vi "Marvin.vi"() -> ()   [LabVIEW 2017]
uses:
  Marvin ATP Remake 1.5.18/PCAN_Driver/ControlCAN.llb/CAN Channel.ctl
  Marvin ATP Remake 6.5.18 - Copy/PCAN_Driver/ControlCAN.llb/DevType.ctl
  Marvin ATP Remake 6.5.18/PCAN_Driver/ControlCAN.llb/VCI_INIT_CONFIG.ctl
  Marvin ATP Remake 6.5.18/PCAN_Driver/ControlCAN.llb/InitFlag.ctl
  Marvin ATP Remake 6.5.18/PCAN_Driver/ControlCAN.llb/Fliter.ctl
  Marvin ATP Remake 6.5.18/PCAN_Driver/ControlCAN.llb/Mode.ctl
  <vilib>/Utility/miscctls.llb/LVMinMaxIncTypeDef.ctl
  PCAN_Driver/ControlCAN.llb/VCI_CAN_OBJ.ctl
  PCAN_Driver/ControlCAN.lvlib
panel:
  in  "Graph Plot":bool
  in  "Get":bool
  in  "Set":bool
  out "Array 2":dbl[](array[numeric])
  in  "Clear Data Array":bool
  in  "PlayPause Data Array":bool
  out "CAN Data":cluster{"Frame Data":u64, "Frame ID":u32}[](array[cluster]) {"Frame ID" format="%.0x"; "Frame Data" format="%016x"}
  out "Waveform Chart":dbl(graph)
  in  "Help Button":bool
  in  "Clear Monitor":bool
  out "Array":u64[][](array[numeric]) format="%016x"
  out "Ambient Over temp":bool
  out "Ambient Sensor temp":bool
  out "Ambient Temperature":dbl
  in  "Motor Over Temp":bool
  in  "Speed control":bool
  out "Unit Adress":string
  in  "Serial Send":bool
  in  "Index":u16(ring) items=["1"=1, "2"=2, "3"=3]
  out "read buffer":string
  in  "SetGet":enum16{"Get", "Set"}(ring)
  in  "Function":T1(ring)
  in  "Value":dbl
  in  "Value 1/2":enum16{"1", "2"}(ring)
  out "Msg Count":u32
  in  "Param to Set":u16(ring) items=["EBAY 5F"=95, "AHU 3F"=63, "AHU 2F"=47]
  out "UUT":u8
  out "Horizontal Progress Bar":i32(slide) min=0 max=48 scale=0.0..50.0
  in  "Set Param.":bool
  in  "Serial Monitor":bool caption="Graph Button"
  in  "Serial Com":bool
  in  "VISA resource name":refnum<visa-resource-name>="COM6"
  out "Serial Status":bool
  in  "Graph Button":bool
  in  "Refresh Button":bool
  out "Data Send":u64 format="%016x"
  in  "Motor Speed RPM":u16
  out "Under voltage/Over voltage":bool
  out "Speed error":bool
  out "Derated drive temp":bool
  out "Motor Over temperature":bool
  out "Commutation err":bool
  out "Motor Sensor temp Fauilre":bool
  out "Drive Over temperature":bool
  out "Drive Sensor temp Failure":bool
  out "Motor Phase Current RMS":dbl
  out "ECS State":u16
  out "Motor Speed RPM":dbl
  out "Motor Stator Temp.":dbl
  out "Power transistor Heat sink Temp.":dbl
  out "DC Current":dbl
  out "DC Voltage":dbl
  in  "Can Send":bool
  in  "Stop":bool
  out "Config_CANAT":T8 {"DevType" items=["USB-CAN"=3, "USB-CAN2"=4]; "CanIndex" items=["通道1", "通道2"]; "VCI_INIT_CONFIG"."Fliter" items=["接收所有类型"=3, "只接收标准帧"=4, "只接收扩展帧"=7]; "VCI_INIT_CONFIG"."Mode" items=["正常工作", "自测模式（环回）", "仅侦听模式"]; "VCI_INIT_CONFIG"."InitFlag" items=["使用Flash参数", "使用界面设置参数"]}
  in  "Channel 2":T3 caption="Channel" items=["Channel 1", "Channel 2"]
  out "CAN Status":bool
  out "Driver Version":string
  out "Hall Sensor Fault":bool
  out "Motor Phase Current":dbl
  in  "Motor Phase Current":u16
  # "ver 1.7e"
  # "Marvin"
  # "REDLER TECHNOLOGIES LTD"
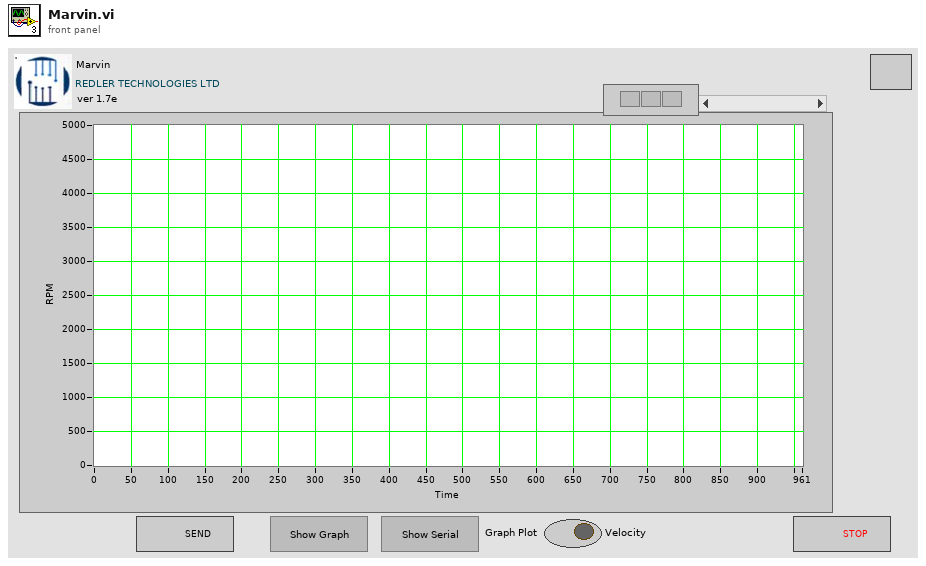
[diagram p1: front panel]
types:
  T1 = enum16{"Enable Conf. EP=1", "Serial Number", "Temperature", "Unit Adress", "Calibration", "Velocity", "Version"}
  T2 = typedef "ControlCAN.lvlib/DevType.ctl" = u32
  T3 = typedef "ControlCAN.lvlib/CAN Channel.ctl" = u32
  T4 = typedef "ControlCAN.lvlib/VCI_INIT_CONFIG.ctl" = cluster{"AccCode":u32, "AccMask":u32, "InitFlag":T5, "Fliter":T6, "Timing0":u8, "Timing1":u8, "Mode":T7}
  T5 = typedef "ControlCAN.lvlib/InitFlag.ctl" = u32
  T6 = typedef "ControlCAN.lvlib/Fliter.ctl" = u8
  T7 = typedef "ControlCAN.lvlib/Mode.ctl" = u8
  T8 = cluster{"DevType":T2, "DevIndex":u32, "CanIndex":T3, "VCI_INIT_CONFIG":T4}
  T9 = cluster{"ID":u32, "MSGTYPE":u8, "LEN":u8, "aDATA":u8[]}[]
  T10 = cluster{"ID":u32, "MSGTYPE":u8, "LEN":u8, "aDATA":u8[]}
  T11 = enum8{"Enabled", "Disabled", "Disabled and Grayed Out"}
  T12 = typedef "LVMinMaxIncTypeDef.ctl" = cluster{"Minimum":dbl, "Maximum":dbl, "Increment":dbl}
  T13 = enum32{"Invalid", "Standard", "Closed", "Hidden", "Minimized", "Maximized"}
  T14 = typedef "ControlCAN.lvlib/VCI_CAN_OBJ.ctl" = cluster{"ID":u32, "TimeStamp":u32, "TimeFlag":u8, "SendType":u8, "RemoteFlag":u8, "ExternFlag":u8, "DataLen":u8, "Data":u8[], "Reserved":u8[]}
  T15 = cluster{"Type":enum16{"接收", "发送"}, "Channel":T3, "Time":timestamp, "VCI_CAN_OBJ":T14}[]
  T16 = cluster{"Type":enum16{"接收", "发送"}, "Channel":T3, "Time":timestamp, "VCI_CAN_OBJ":T14}
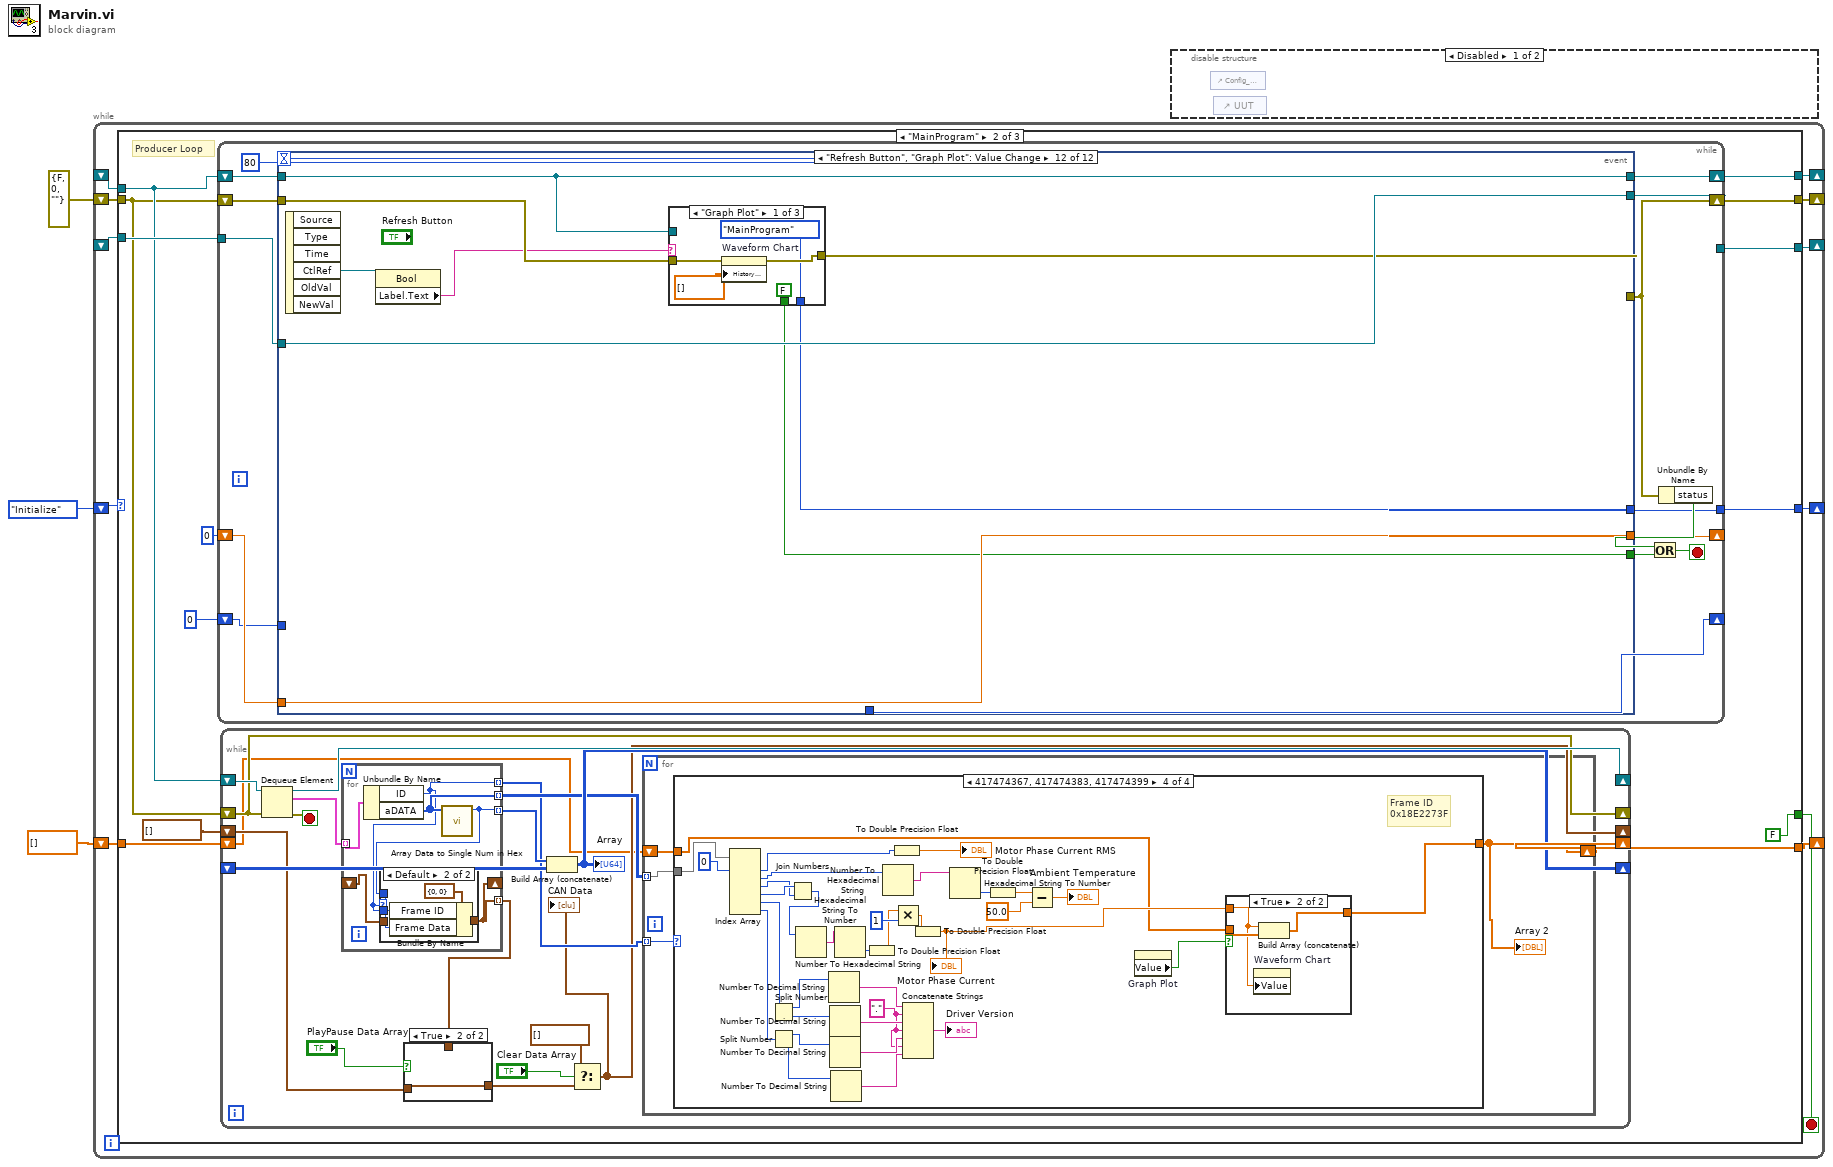
[diagram p0: block diagram]
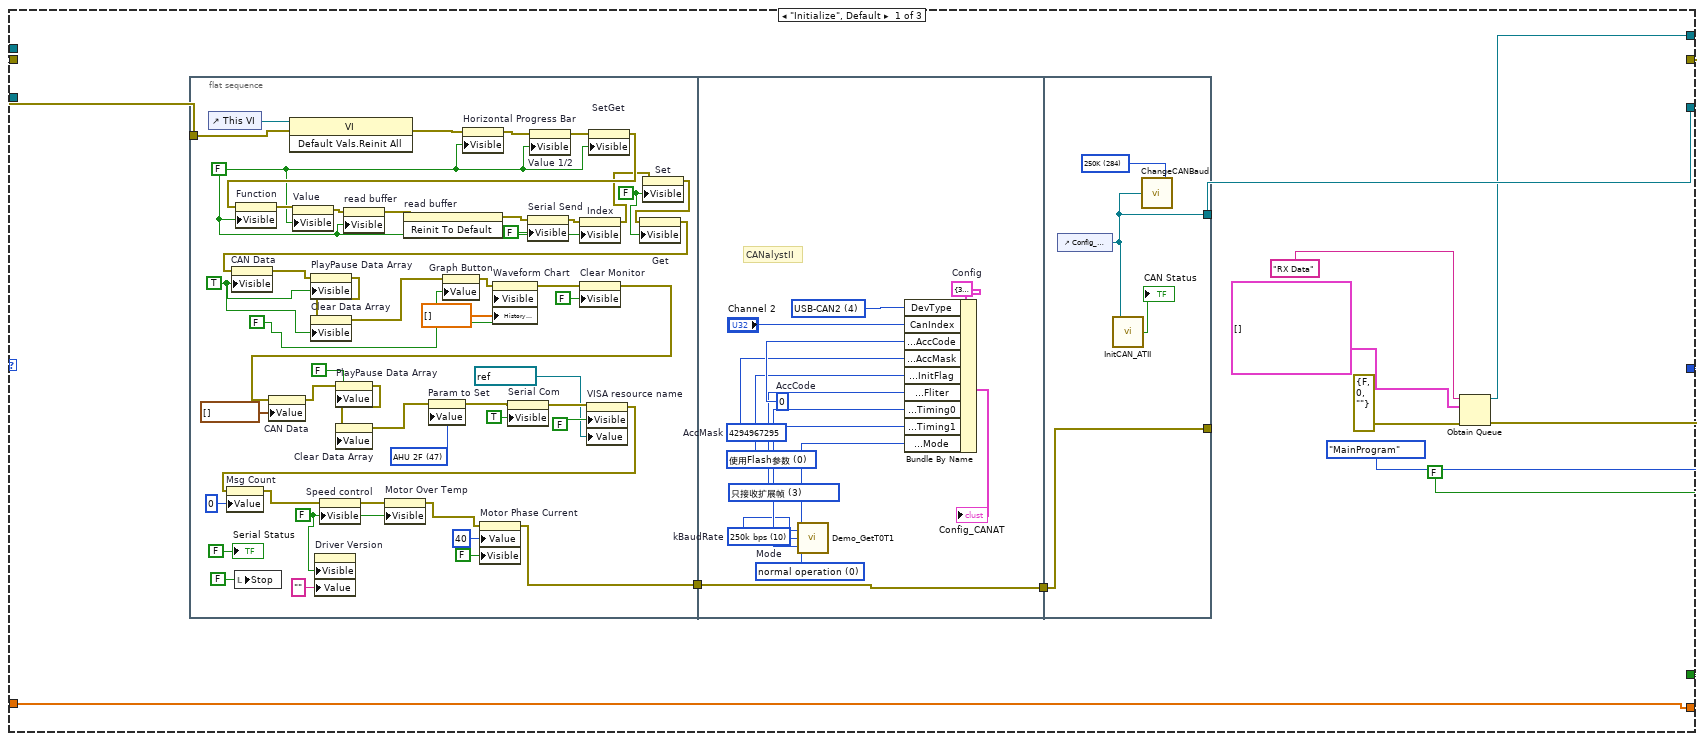
[diagram p3: hidden frame]
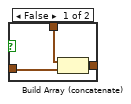
[diagram p4: hidden frame]
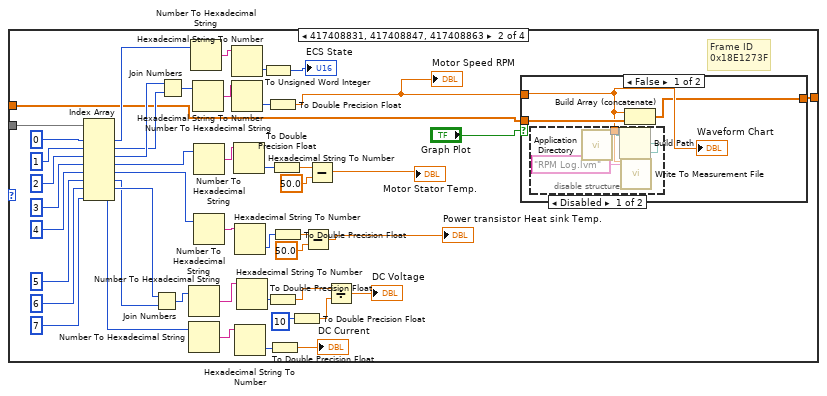
[diagram p6: hidden frame]
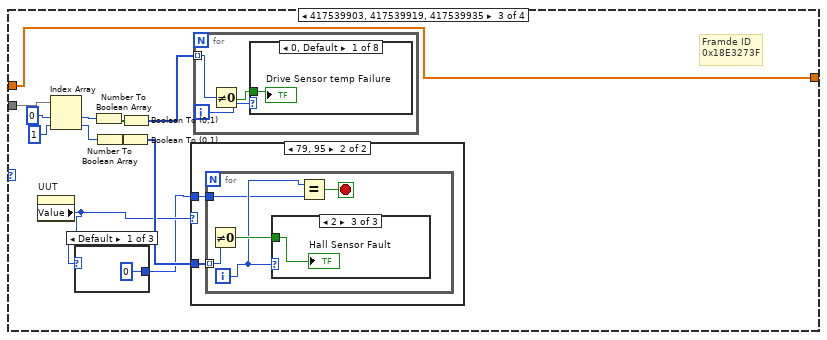
[diagram p9: hidden frame]
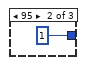
[diagram p10: hidden frame]
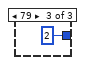
[diagram p11: hidden frame]
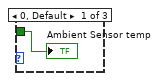
[diagram p13: hidden frame]
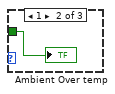
[diagram p14: hidden frame]
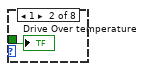
[diagram p15: hidden frame]
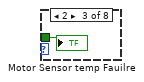
[diagram p16: hidden frame]
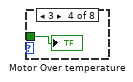
[diagram p17: hidden frame]
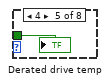
[diagram p18: hidden frame]
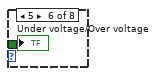
[diagram p19: hidden frame]
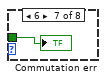
[diagram p20: hidden frame]
diagram:
  n1 = while {
    shift-right: [w9] -> _
    shift-left: enum16{"Stop", "MainProgram", "Initialize"}."Initialize" -> [w14]
    shift-right: [w13] -> _
    shift-left: _ -> [w12]
    shift-right: [w11] -> _
    shift-left: _ -> [w8]
    shift-right: [w10] -> _
    shift-left: errorcluster {"status"=FALSE, "code"=0, "source"=""} ("error out") -> [w7]
    shift-right: [w4] -> _
    shift-left: dbl[] [] -> [w5]
    stop <- w6 stop-if-true
    n2 = case shown="\"MainProgram\"" w14 {
      tunnel: [w26 w103 w1075] -> w13
      tunnel: w12 -> [_ w106 w1075]
      tunnel: [w22 w105 w1076] -> w11
      tunnel: [w21 w104 w1077] -> w10
      tunnel: [enum16{"Stop", "MainProgram", "Initialize"}."MainProgram" w102 enum16{"Stop", "MainProgram", "Initialize"}."Stop"] -> w9
      tunnel: w8 -> [_ w101 w1076]
      tunnel: w7 -> [w19 w100 w1078]
      tunnel: [FALSE ("Stop") FALSE ("Stop") w1074] -> w6
      tunnel: w5 -> [w15 w97 w1072]
      tunnel: [w15 w96 w1072] -> w4
      frame "Initialize", Default {
        n3 = flat-sequence {
          tunnel: w19 -> [w58]
          tunnel: [w34] -> w17
          tunnel: [w77] -> w18
          tunnel: w17 -> [w77]
          tunnel: [w91] -> w26
          tunnel: w18 -> [w90]
          tunnel: [w90] -> _
          frame #0 {
            w31 = FALSE ("Visible")
            w43 = FALSE ("PlayPause Data Array")
            w37 = FALSE ("Visible")
            w68 = u16 47 items=["EBAY 5F"=95, "AHU 3F"=63, "AHU 2F"=47] ("Param to Set")
            w38 = TRUE ("Visible")
            w52 = FALSE ("Visible")
            w42 = FALSE ("Graph Button")
            n4 = control-ref of="This VI"() -> (w76:refnum<vi>)
            n5 = local write "Stop"(FALSE ("Stop")) -> ()
            n6 = invoke class="VI" method="Default Vals.Reinit All"(reference=w76, error in=w58) -> (error out=w57:errorcluster)  [unwired: 1 in, 2 out]
            n7 = property on="Driver Version" class="Str"("Visible"=w37, "Value"="" ("Driver Version")) -> ()  [unwired: 2 in, 2 out]
            n8 = property on="Horizontal Progress Bar" class="Slide (strict)"(error in=w57, "Visible"=w52) -> (error out=w66:errorcluster)  [unwired: 1 in, 1 out]
            n9 = property on="Value 1/2" class="Enum (strict)"(error in=w66, "Visible"=w52) -> (error out=w65:errorcluster)  [unwired: 1 in, 1 out]
            n10 = property on="SetGet" class="Enum (strict)"(error in=w65, "Visible"=w52) -> (error out=w64:errorcluster)  [unwired: 1 in, 1 out]
            n11 = property on="Function" class="Enum (strict)"(error in=w64, "Visible"=w52) -> (error out=w63:errorcluster)  [unwired: 1 in, 1 out]
            n12 = property on="Value" class="DigNum (strict)"(error in=w63, "Visible"=w52) -> (error out=w62:errorcluster)  [unwired: 1 in, 1 out]
            n13 = property on="read buffer" class="Str"(error in=w62, "Visible"=w52) -> (error out=w54:errorcluster)  [unwired: 1 in, 1 out]
            n14 = invoke on="read buffer" class="Str" method="Reinit To Default"(error in=w54) -> (error out=w53:errorcluster)  [unwired: 2 in, 2 out]
            n15 = property on="Serial Send" class="Bool (strict)"(error in=w53, "Visible"=FALSE) -> (error out=w61:errorcluster)  [unwired: 1 in, 1 out]
            n16 = property on="Index" class="Ring (strict)"(error in=w61, "Visible"=w52) -> (error out=w29:errorcluster)  [unwired: 1 in, 1 out]
            n17 = property on="Set" class="Bool (strict)"(error in=w29, "Visible"=w31) -> (error out=w30:errorcluster)  [unwired: 1 in, 1 out]
            n18 = property on="Get" class="Bool (strict)"(error in=w30, "Visible"=w31) -> (error out=w28:errorcluster)  [unwired: 1 in, 1 out]
            n19 = property on="CAN Data" class="Arr (strict)"(error in=w28, "Visible"=w38) -> (error out=w41:errorcluster)  [unwired: 1 in, 1 out]
            n20 = property on="PlayPause Data Array" class="Bool (strict)"(error in=w41, "Visible"=w38) -> (error out=w40:errorcluster)  [unwired: 1 in, 1 out]
            n21 = property on="Clear Data Array" class="Bool (strict)"(error in=w40, "Visible"=w38) -> (error out=w39:errorcluster)  [unwired: 1 in, 1 out]
            n22 = property on="Graph Button" class="Bool (strict)"(error in=w39, "Value"=w42) -> (error out=w50:errorcluster)  [unwired: 1 in, 1 out]
            n23 = property on="Waveform Chart" class="WFChart (strict)"(error in=w50, "Visible"=w42, "History Data"=dbl[] [] ("Waveform Chart")) -> (error out=w49:errorcluster)  [unwired: 1 in, 1 out]
            n24 = property on="Clear Monitor" class="Bool"(error in=w49, "Visible"=FALSE) -> (error out=w48:errorcluster)  [unwired: 1 in, 1 out]
            n25 = property on="CAN Data" class="Arr (strict)"(error in=w48, "Value"=cluster{"Frame Data":u64, "Frame ID":u32}[] [] ("CAN Data")) -> (error out=w46:errorcluster)  [unwired: 1 in, 1 out]
            n26 = property on="PlayPause Data Array" class="Bool (strict)"(error in=w46, "Value"=w43) -> (error out=w45:errorcluster)  [unwired: 1 in, 1 out]
            n27 = property on="Clear Data Array" class="Bool (strict)"(error in=w45, "Value"=w43) -> (error out=w44:errorcluster)  [unwired: 1 in, 1 out]
            n28 = property on="Param to Set" class="Ring (strict)"(error in=w44, "Value"=w68) -> (error out=w60:errorcluster)  [unwired: 1 in, 1 out]
            n29 = property on="Serial Com" class="Bool"(error in=w60, "Visible"=TRUE) -> (error out=w73:errorcluster)  [unwired: 1 in, 1 out]
            n30 = property on="VISA resource name" class="VISAName"(error in=w73, "Visible"=FALSE, "Value"=refnum<visa-resource-name> "COM1" ("VISA resource name")) -> (error out=w59:errorcluster)  [unwired: 1 in, 1 out]
            n31 = property on="Msg Count" class="DigNum (strict)"(error in=w59, "Value"=u32 0 ("Msg Count")) -> (error out=w56:errorcluster)  [unwired: 1 in, 1 out]
            n32 = property on="Speed control" class="Bool (strict)"(error in=w56, "Visible"=w37) -> (error out=w55:errorcluster)  [unwired: 1 in, 1 out]
            n33 = property on="Motor Over Temp" class="Bool (strict)"(error in=w55, "Visible"=w37) -> (error out=w35:errorcluster)  [unwired: 1 in, 1 out]
            n34 = property on="Motor Phase Current" class="DigNum (strict)"(error in=w35, "Value"=u16 40 ("Motor Phase Current"), "Visible"=FALSE) -> (error out=w34:errorcluster)  [unwired: 1 in, 1 out]
            "Serial Status" <- FALSE ("Serial Status")
          }
          frame #1 {
            w81 = u32 4294967295  # AccMask
            w80 = T5 0 items=["使用Flash参数", "使用界面设置参数"] ("InitFlag")
            w78 = T7 0 items=["normal operation", "Listen-only mode", "test mode"]  # Mode
            w79 = T6 3 items=["接收所有类型"=1, "只接收标准帧"=2, "只接收扩展帧"=3] ("Fliter")
            w85 = u8 10 items=["5k bps"=1, "10k bps"=2, "20k bps"=3, "40k bps"=4, "50k bps"=5, "80k bps"=6, "100k bps"=7, "125k bps"=8, "200k bps"=9, "250k bps"=10, "400k bps"=11, "500k bps"=12, "666k bps"=13, "800k bps"=14, "1000k bps"=15, "33.33k bps"=16, "66.66k bps"=17, "83.33k bps"=18]  # kBaudRate
            w82 = u32 0  # AccCode
            w83 = T2 4 items=["USB-CAN"=3, "USB-CAN2"=4] ("DevType")
            w84 = T8 {"DevType"=3, "DevIndex"=0, "CanIndex"=0, "VCI_INIT_CONFIG"={"AccCode"=0, "AccMask"=0, "InitFlag"=1, "Fliter"=7, "Timing0"=0, "Timing1"=0, "Mode"=0}}  # Config
            # "CANalystII"
            n35 = call "Demo_GetT0T1.vi"("kBaudRate"=w85) -> ("Timing0"=w87:u8, "Timing1"=w88:u8)
            n36 = Bundle By Name(cluster=w84, "DevType"=w83, "CanIndex"="Channel 2", "VCI_INIT_CONFIG.AccCode"=w82, "VCI_INIT_CONFIG.AccMask"=w81, "VCI_INIT_CONFIG.InitFlag"=w80, "VCI_INIT_CONFIG.Fliter"=w79, "VCI_INIT_CONFIG.Timing0"=w87, "VCI_INIT_CONFIG.Timing1"=w88, "VCI_INIT_CONFIG.Mode"=w78) -> (→"Config_CANAT":T8)
          }
          frame #2 {
            w92 = u16 284 items=["1M"=20, "500K"=28, "250K"=284, "125K"=796, "100K"=17199, "50K"=18223, "20K"=21295, "10K"=26415, "5K"=32639] ("baud in")
            n37 = control-ref of="Config_CANAT"() -> (w91:refnum<vi>)
            n38 = call "InitCAN_ATII.vi"("Config"=w91) -> ("Sts"=→"CAN Status":bool)
            n39 = call "ChangeCANBaud.vi"("baud in"=w92, "reference"=w91) -> ()
          }
        }
        n40 = Obtain Queue(name (unnamed)="RX Data", element data type=T9 [], error in (no error)=errorcluster {"status"=FALSE, "code"=0, "source"=""}) -> (queue out=w22:refnum<queue>, error out=w21:errorcluster)  [unwired: 2 in, 1 out]
      }
      frame "MainProgram" {
        # "Producer Loop"
        n41 = while {
          shift-right: [w283] -> w104
          shift-left: w100 -> [w285]
          shift-right: [w284] -> w105
          shift-left: w101 -> [w286]
          tunnel: w106 -> [w287]
          tunnel: [w280] -> w103
          tunnel: [w279] -> w102
          shift-right: [w277] -> _
          shift-left: 0 -> [w278]
          shift-right: [w275] -> _
          shift-left: 0 -> [w276]
          stop <- w288 stop-if-true
          n42 = event shown="[11] \"Refresh Button\", \"Graph Plot\": Value Change" {
            selector: _ -> [_ _ _ _ _ _ _ _ _ _ _ _]
            dyn-events: _ -> [_ _ _ _ _ _ _ _ _ _ _ _]
            timeout: 80 ("Numeric") -> [_ _ _ _ _ _ _ _ _ _ _ _]
            tunnel: w287 -> [w309 w387 w408 w495 w777 w875 w898 w997 w1017 w1034 w1049 w1058]
            tunnel: w286 -> [w306 w388 w411 w496 w776 w876 w919 w998 w1016 w1035 w1046 w1056]
            tunnel: w285 -> [w291 w386 w406 w472 w769 w868 w918 w978 w1012 w1027 w1045 w1057]
            tunnel: [w304 w388 w411 w496 w776 w876 w919 w998 w1016 w1035 w1044 w1056] -> w284
            tunnel: [w303 w381 w407 w488 w765 w865 w918 w985 w1009 w1025 w1042 w1055] -> w283
            tunnel: [FALSE ("Stop") FALSE ("Stop") FALSE ("Stop") FALSE ("Stop") FALSE ("Stop") FALSE ("Stop") FALSE ("Stop") FALSE ("Stop") FALSE ("Stop") FALSE ("Stop") TRUE ("Stop") w1051] -> w281
            tunnel: [w302 w387 w408 w495 w777 w875 w898 w997 w1017 w1034 w1049 w1058] -> w280
            tunnel: [enum16{"Stop", "MainProgram", "Initialize"}."MainProgram" enum16{"Stop", "MainProgram", "Initialize"}."MainProgram" enum16{"Stop", "MainProgram", "Initialize"}."MainProgram" enum16{"Stop", "MainProgram", "Initialize"}."MainProgram" enum16{"Stop", "MainProgram", "Initialize"}."MainProgram" enum16{"Stop", "MainProgram", "Initialize"}."MainProgram" enum16{"Stop", "MainProgram", "Initialize"}."MainProgram" enum16{"Stop", "MainProgram", "Initialize"}."MainProgram" enum16{"Stop", "MainProgram", "Initialize"}."MainProgram" enum16{"Stop", "MainProgram", "Initialize"}."MainProgram" enum16{"Stop", "MainProgram", "Initialize"}."Stop" w1050] -> w279
            tunnel: w278 -> [w298 w391 w404 w484 w767 w879 w884 w993 w1008 w1023 w1041 w1054]
            tunnel: [w297 w391 w404 w484 w767 w879 w884 w993 w1008 w1023 w1041 w1054] -> w277
            tunnel: w276 -> [w290 _ _ _ _ _ _ _ _ _ _ _]
            tunnel: [w290 _ _ _ _ _ _ _ _ _ _ _] -> w275
            event Timeout {
              n43 = event-data() -> ()  [unwired: 1 in, 3 out]
              n44 = property class="Clust (strict)"(reference=w309) -> (reference out=w302:refnum<vi>, "Value"=w310:T8)  [unwired: 1 in, 1 out]
              n45 = property on="Speed control" class="Bool (strict)"(error in=w291) -> ("Value"=w292:bool)  [unwired: 1 in, 2 out]
              n46 = case shown="True" w292 {
                frame False {
                }
                frame True {
                  n47 = property on="Motor Speed RPM" class="DigNum (strict)"() -> ("Value"=w316:u16)  [unwired: 2 in, 2 out]
                  n48 = control-ref of="Config_CANAT"() -> (w315:refnum<vi>)
                  n49 = control-ref of="UUT"() -> (w314:refnum<vi>)
                  n50 = call "CANSendMotorSpeed.vi"("Remote"=TRUE, "Motor Speed RPM"=w316, "UUT"=w314, "CAN Cluster in"=w315) -> ()  [unwired: 7 in, 1 out]
                }
              }
              n51 = Unbundle By Name(w310) -> ("DevType"=w311:T2, "CanIndex"=w307:T3)
              n52 = property on="Horizontal Progress Bar" class="Slide (strict)"(error in=w291, "Visible"=FALSE) -> (error out=w293:errorcluster)  [unwired: 1 in, 1 out]
              n53 = call "VCI_Receive.vi"("CANIndex"=w307, "DevIndex"=u32 0, "DevType"=w311) -> ("Recieve"=w305:T14[])  [unwired: 3 in, 5 out]
              n54 = Empty Array?(array=w305) -> (empty?=w308:bool)
              n55 = case shown="False" w308 {
                tunnel: w307 -> [w328 _]
                tunnel: w302 -> [w326 _]
                tunnel: w306 -> [w325 w380]
                tunnel: w293 -> [w324 w379]
                tunnel: w305 -> [w329 _]
                tunnel: [w319 w379] -> w303
                tunnel: [w318 w380] -> w304
                tunnel: [w317 0] -> w294
                frame False {
                  n56 = call "Demo_MakeDispBuff.vi"("Channel"=w328, "Type"=enum16{"接收", "发送"}."接收", "OBJs"=w329) -> ("Buffer"=w327:T15)
                  n57 = for {
                    N: 3 -> [_]
                    tunnel: w327 -> [w343]
                    tunnel: w326 -> [w342]
                    tunnel: w325 -> [w333]
                    tunnel: w324 -> [w332]
                    tunnel: [w335] -> w322 mode=indexing
                    tunnel: [w333] -> w321
                    tunnel: [w332] -> w320
                    tunnel: [w331] -> w317
                    i -> [w331]
                    n58 = property class="Clust (strict)"(reference=w342) -> ("Value"=w340:T8)  [unwired: 1 in, 2 out]
                    n59 = Index Array(array=w343, index=w331) -> (element=w336:T16)
                    n60 = Unbundle By Name(w336) -> ("Channel"=w338:T3, "VCI_CAN_OBJ"=w341:T14)  [unwired: 2 out]
                    n61 = Unbundle By Name(w340) -> ("CanIndex"=w339:T3)
                    n62 = Equal?(x=w339, y=w338) -> (x = y?=w337:bool)
                    n63 = case shown="True" w337 {
                      tunnel: w341 -> [_ w359]
                      tunnel: [w344 w355] -> w335
                      tunnel: T10 {"ID"=0, "MSGTYPE"=0, "LEN"=0, "aDATA"=[]} ("Msg") -> [w344 w354]
                      frame False {
                      }
                      frame True {
                        n64 = Unbundle By Name(w359) -> ("ID"=w353:u32, "DataLen"=w358:u8, "Data"=w356:u8[])
                        n65 = Bundle By Name(cluster=w354, "ID"=w353, "MSGTYPE"=u8 0, "LEN"=w358, "aDATA"=w356) -> (w355:T10)
                        n66 = Unbundle By Name(w355) -> ("ID"=w351:u32)
                        n67 = Split Number(x=w351) -> (lo(x)=w352:u16)  [unwired: 1 out]
                        n68 = Split Number(x=w352) -> (lo(x)=w349:u8)  [unwired: 1 out]
                        "UUT" <- w349
                        n69 = case shown="95" w349 {
                          tunnel: ["EBAY 5F" "PUMP 4F" w372 "AHU 3F" "AHU 2F"] -> w348
                          tunnel: [TRUE w369 w373 w374 w376] -> w346
                          tunnel: [FALSE w369 w371 w374 w376] -> w345
                          frame 95 {
                          }
                          frame 79 {
                            w369 = TRUE
                          }
                          frame Default {
                            n70 = property on="Hall Sensor Fault" class="Bool (strict)"() -> ("Visible"=w371:bool)  [unwired: 2 in, 2 out]
                            n71 = property on="Speed control" class="Bool (strict)"() -> ("Visible"=w373:bool)  [unwired: 2 in, 2 out]
                            n72 = property on="Unit Adress" class="Str"() -> ("Value"=w372:string)  [unwired: 2 in, 2 out]
                          }
                          frame 63 {
                            w374 = FALSE
                          }
                          frame 47 {
                            w376 = FALSE
                          }
                        }
                        n73 = Not Equal To 0?(x=w349) -> (x != 0?=w350:bool)
                        n74 = case shown="True" w350 {
                          tunnel: w349 -> [_ w365]
                          tunnel: w348 -> [_ w362]
                          tunnel: [w360 w361] -> w347
                          frame False {
                            n75 = property on="Unit Adress" class="Str"() -> ("Value"=w360:string)  [unwired: 2 in, 2 out]
                          }
                          frame True {
                            n76 = Number To Decimal String(number=w365) -> (decimal integer string=w364:string)  [unwired: 1 in]
                            n77 = call <vilib>:"Space Constant.vi"() -> ("String"=w363:string)
                            n78 = Concatenate Strings(w364, w363, w362) -> (w361:string)
                          }
                        }
                        "Unit Adress" <- w347
                        n79 = property on="Driver Version" class="Str"("Visible"=w346) -> ()  [unwired: 2 in, 2 out]
                        n80 = property on="Hall Sensor Fault" class="Bool (strict)"("Visible"=w345) -> ()  [unwired: 2 in, 2 out]
                        n81 = property on="Motor Phase Current" class="DigNum (strict)"("Visible"=w345) -> ()  [unwired: 2 in, 2 out]
                        n82 = property on="Motor Phase Current" class="DigNum (strict)"("Visible"=w345) -> ()  [unwired: 2 in, 2 out]
                        n83 = property on="Ambient Over temp" class="Bool (strict)"("Visible"=w346) -> ()  [unwired: 2 in, 2 out]
                        n84 = property on="Ambient Sensor temp" class="Bool (strict)"("Visible"=w346) -> ()  [unwired: 2 in, 2 out]
                        n85 = property on="Ambient Temperature" class="DigNum (strict)"("Visible"=w346) -> ()  [unwired: 2 in, 2 out]
                        n86 = property on="Motor Over Temp" class="Bool (strict)"("Visible"=w346) -> ()  [unwired: 2 in, 2 out]
                        n87 = property on="Speed control" class="Bool (strict)"("Visible"=w346) -> ()  [unwired: 2 in, 2 out]
                      }
                    }
                  }
                  n88 = Enqueue Element(queue=w321, element=w322, error in (no error)=w320) -> (queue out=w318:refnum<queue>, error out=w319:errorcluster)  [unwired: 2 out]
                }
                frame True {
                }
              }
              n89 = Divide(x=w294, y=u32 2) -> (x/y=w295:dbl)
              n90 = Add(x=w295, y=w298) -> (x+y=w297:dbl)
              "Msg Count" <- w297
            }
            event "Clear Monitor": Value Change {
              n91 = event-data() -> ()  [unwired: 1 in, 6 out]
              n92 = property on="VISA resource name" class="VISAName"(error in=w386) -> (error out=w385:errorcluster, "Value"=w384:refnum<visa-resource-name>)  [unwired: 1 in, 1 out]
              n93 = disable-structure shown="Enabled" {
                disable-tunnel: w385 -> [w396 w399]
                disable-tunnel: w384 -> [w394 w400]
                disable-tunnel: [w393 ""] -> w383
                disable-tunnel: [w392 w398] -> w382
                frame Disabled {
                  n94 = call "Serial.vi"("error in (no error)"=w396, "Clear Log"=TRUE, "VISA resource name"=w394) -> ("error out"=w392:errorcluster, "read buffer"=w393:string)  [unwired: 7 in]
                }
                frame Enabled {
                  n95 = VISA Flush I/O Buffer(VISA resource name=w400, error in (no error)=w399) -> (error out=w398:errorcluster)  [unwired: 1 in, 1 out]
                }
              }
              n96 = property on="read buffer" class="Str"(error in=w382, "Value"=w383) -> (error out=w381:errorcluster)  [unwired: 1 in, 1 out]
            }
            event "Serial Monitor": Value Change {
              n97 = event-data() -> ()  [unwired: 1 in, 6 out]
              n98 = property on="Serial Status" class="Bool (strict)"(error in=w406) -> (error out=w405:errorcluster, "Value"=w403:bool)  [unwired: 1 in, 1 out]
              n99 = Or(x=FALSE, y=w403) -> (x .or. y?=w402:bool)
              n100 = case shown="True" w402 {
                tunnel: w405 -> [w415 w434]
                tunnel: [w413 w439] -> w407
                frame False {
                  n101 = call "Display Message to User3"("error in (no error)"=w415) -> ("error out"=w414:errorcluster)  [unwired: 9 in, 1 out]
                  n102 = property on="Serial Monitor" class="Bool (strict)"(error in=w414, "Value"=FALSE ("Serial Monitor")) -> (error out=w413:errorcluster)  [unwired: 1 in, 1 out]
                }
                frame True {
                  w422 = FALSE ("Visible")
                  w427 = FALSE ("Visible")
                  w436 = FALSE ("Visible")
                  w437 = u16 1 items=["1"=1, "2"=2, "3"=3] ("Index")
                  n103 = property on="Index" class="Ring (strict)"(error in=w434, "Value"=w437) -> (error out=w433:errorcluster)  [unwired: 1 in, 1 out]
                  n104 = property on="Value 1/2" class="Enum (strict)"(error in=w433, "Visible"=w436) -> (error out=w432:errorcluster)  [unwired: 1 in, 1 out]
                  n105 = property on="Value" class="DigNum (strict)"(error in=w432, "Visible"=w436) -> (error out=w431:errorcluster)  [unwired: 1 in, 1 out]
                  n106 = property on="SetGet" class="Enum (strict)"(error in=w431, "Value"=enum16{"Get", "Set"}."Get" ("SetGet")) -> (error out=w420:errorcluster)  [unwired: 1 in, 1 out]
                  n107 = property on="Set" class="Bool (strict)"(error in=w420, "Visible"=w422) -> (error out=w421:errorcluster)  [unwired: 1 in, 1 out]
                  n108 = property on="Get" class="Bool (strict)"(error in=w421, "Visible"=w422) -> (error out=w419:errorcluster)  [unwired: 1 in, 1 out]
                  n109 = property on="Serial Send" class="Bool (strict)"(error in=w419, "Visible"=w427) -> (error out=w426:errorcluster)  [unwired: 1 in, 1 out]
                  n110 = property on="Clear Monitor" class="Bool"(error in=w426, "Visible"=w427) -> (error out=w425:errorcluster)  [unwired: 1 in, 1 out]
                  n111 = property on="Function" class="Enum (strict)"(error in=w425, "Value"=T1."Serial Number" ("Function")) -> (error out=w430:errorcluster)  [unwired: 1 in, 1 out]
                  n112 = property on="Index" class="Ring (strict)"(error in=w430, "DisabledEnum"=T11."Disabled and Grayed Out" ("Disabled")) -> (error out=w428:errorcluster)  [unwired: 1 in, 1 out]
                  n113 = case shown="True" "Serial Monitor" {
                    selector: "Serial Monitor" -> [w445 w467]
                    tunnel: w428 -> [w444 w463]
                    tunnel: [w446 w464] -> w439
                    tunnel: [w440 TRUE] -> w424
                    tunnel: [FALSE ("Visible") TRUE ("Visible")] -> w417
                    tunnel: [w440 FALSE ("Visible")] -> w416
                    frame False {
                      w440 = FALSE
                      n114 = property on="Graph Button" class="Bool (strict)"(error in=w444) -> (error out=w443:errorcluster, "Value"=w442:bool)  [unwired: 1 in, 1 out]
                      n115 = case shown="True" w442 {
                        tunnel: [w450 w455] -> w447
                        tunnel: w443 -> [w452 w458]
                        tunnel: w445 -> [w453 _]
                        frame False {
                          n116 = property on="Waveform Chart" class="WFChart (strict)"(error in=w452, "Visible"=FALSE) -> (error out=w449:errorcluster)  [unwired: 1 in, 1 out]
                          n117 = Not(x=w453) -> (.not. x?=w448:bool)
                          n118 = property on="PlayPause Data Array" class="Bool (strict)"("Visible"=w448) -> ()  [unwired: 2 in, 2 out]
                          n119 = property on="Clear Data Array" class="Bool (strict)"("Visible"=w448) -> ()  [unwired: 2 in, 2 out]
                          n120 = property on="CAN Data" class="Arr (strict)"(error in=w449, "Visible"=w448) -> (error out=w450:errorcluster)  [unwired: 1 in, 1 out]
                        }
                        frame True {
                          w454 = FALSE ("Visible")
                          n121 = property on="Waveform Chart" class="WFChart (strict)"(error in=w458, "Visible"=TRUE) -> (error out=w456:errorcluster)  [unwired: 1 in, 1 out]
                          n122 = property on="PlayPause Data Array" class="Bool (strict)"("Visible"=w454) -> ()  [unwired: 2 in, 2 out]
                          n123 = property on="Clear Data Array" class="Bool (strict)"("Visible"=w454) -> ()  [unwired: 2 in, 2 out]
                          n124 = property on="CAN Data" class="Arr (strict)"(error in=w456, "Visible"=w454) -> (error out=w455:errorcluster)  [unwired: 1 in, 1 out]
                        }
                      }
                      n125 = property on="Serial Monitor" class="Bool (strict)"(error in=w447, "Value"=w445) -> (error out=w446:errorcluster)  [unwired: 1 in, 1 out]
                    }
                    frame True {
                      n126 = Not(x=w467) -> (.not. x?=w461:bool)
                      n127 = property on="PlayPause Data Array" class="Bool (strict)"("Visible"=w461) -> ()  [unwired: 2 in, 2 out]
                      n128 = property on="CAN Data" class="Arr (strict)"(error in=w463, "Visible"=w461) -> (error out=w462:errorcluster)  [unwired: 1 in, 1 out]
                      n129 = property on="Clear Data Array" class="Bool (strict)"("Visible"=w461) -> ()  [unwired: 2 in, 2 out]
                      n130 = property on="Serial Monitor" class="Bool (strict)"(error in=w462, "Value"=w467) -> (error out=w466:errorcluster)  [unwired: 1 in, 1 out]
                      n131 = property on="Graph Button" class="Bool (strict)"(error in=w466, "Value"=w461) -> (error out=w465:errorcluster)  [unwired: 1 in, 1 out]
                      n132 = property on="Waveform Chart" class="WFChart (strict)"(error in=w465, "Visible"=w461) -> (error out=w464:errorcluster)  [unwired: 1 in, 1 out]
                    }
                  }
                  n133 = property on="Index" class="Ring (strict)"("Visible"=w424) -> ()  [unwired: 2 in, 2 out]
                  n134 = property on="SetGet" class="Enum (strict)"("Visible"=w416) -> ()  [unwired: 2 in, 2 out]
                  n135 = property on="Clear Monitor" class="Bool"("Visible"=w424) -> ()  [unwired: 2 in, 2 out]
                  n136 = property on="Function" class="Enum (strict)"("Visible"=w424) -> ()  [unwired: 2 in, 2 out]
                  n137 = property on="Serial Send" class="Bool (strict)"("Visible"=w416) -> ()  [unwired: 2 in, 2 out]
                  n138 = property on="read buffer" class="Str"("Visible"=w424) -> ()  [unwired: 2 in, 2 out]
                  n139 = property on="Set" class="Bool (strict)"("Visible"=w417) -> (error out=w418:errorcluster)  [unwired: 2 in, 1 out]
                  n140 = property on="Get" class="Bool (strict)"(error in=w418, "Visible"=w417) -> ()  [unwired: 1 in, 2 out]
                }
              }
            }
            event "Serial Send", "SetGet", "Set", "Get", "Function": Value Change; "Function": Mouse Move {
              n141 = event-data() -> ("CtlRef"=w483:refnum<vi>)  [unwired: 1 in, 3 out]
              n142 = property class="Ctl"(reference=w483) -> ("Label.Text"=w482:string)  [unwired: 1 in, 2 out]
              n143 = disable-structure shown="Enabled" {
                disable-tunnel: "Function" -> [w502 _]
                disable-tunnel: w472 -> [w501 w529]
                disable-tunnel: [w500 w529] -> w469
                frame Disabled {
                  n144 = case shown="\"Serial Number\"" w502 {
                    tunnel: w501 -> [w504 w509 w516 w518 w521 w525 w527 w528]
                    tunnel: [w503 w511 w515 w520 w523 w524 w527 w528] -> w500
                    frame "Serial Number" {
                      n145 = property on="Index" class="Ring (strict)"(error in=w504, "DisabledEnum"=T11."Disabled and Grayed Out" ("Disabled")) -> (error out=w503:errorcluster)  [unwired: 1 in, 1 out]
                    }
                    frame "Temperature" {
                      n146 = property on="UUT" class="DigNum (strict)"() -> ("Value"=w506:u8)  [unwired: 2 in, 2 out]
                      n147 = case shown="95" w506 {
                        tunnel: [i32[] [2] ("Disabled Items []") i32[] [3] ("Disabled Items []")] -> w507
                        frame 47, 63, Default {
                        }
                        frame 95 {
                        }
                      }
                      n148 = property on="Index" class="Ring (strict)"(error in=w509, "DisabledEnum"=T11."Enabled" ("Disabled"), "Visible"=TRUE, "Disabled Items []"=w507) -> (error out=w511:errorcluster)  [unwired: 1 in, 1 out]
                    }
                    frame "Unit Adress" {
                      n149 = property on="Index" class="Ring (strict)"(error in=w516, "DisabledEnum"=T11."Enabled" ("Disabled"), "Visible"=TRUE) -> (error out=w515:errorcluster)  [unwired: 1 in, 1 out]
                    }
                    frame "Calibration" {
                      n150 = property on="Index" class="Ring (strict)"(error in=w518, "DisabledEnum"=T11."Disabled and Grayed Out" ("Disabled")) -> (error out=w520:errorcluster)  [unwired: 1 in, 1 out]
                    }
                    frame "Velocity" {
                      n151 = property on="Index" class="Ring (strict)"(error in=w521, "DisabledEnum"=T11."Disabled and Grayed Out" ("Disabled")) -> (error out=w523:errorcluster)  [unwired: 1 in, 1 out]
                    }
                    frame "Version" {
                      n152 = property on="Index" class="Ring (strict)"(error in=w525, "DisabledEnum"=T11."Disabled and Grayed Out" ("Disabled")) -> (error out=w524:errorcluster)  [unwired: 1 in, 1 out]
                    }
                    frame "Enable Conf. EP=1" {
                    }
                    frame Default {
                    }
                  }
                }
                frame Enabled {
                }
              }
              n153 = case shown="\"Temperature\"" "Function" {
                tunnel: w469 -> [w533 w537 w541 w545 w549 w553 w555 w557]
                tunnel: [FALSE TRUE TRUE FALSE FALSE FALSE w554 w556] -> w475
                tunnel: [TRUE FALSE TRUE FALSE TRUE FALSE w554 w556] -> w476
                tunnel: [FALSE FALSE FALSE TRUE FALSE FALSE w554 w556] -> w471
                tunnel: [w533 w537 w541 w545 w549 w553 w555 w557] -> w478
                frame "Serial Number" {
                }
                frame "Temperature" {
                }
                frame "Unit Adress" {
                }
                frame "Calibration" {
                }
                frame "Velocity" {
                }
                frame "Version" {
                }
                frame "Enable Conf. EP=1" {
                  w554 = FALSE
                }
                frame Default {
                  w556 = FALSE
                }
              }
              n154 = property on="Index" class="Ring (strict)"(error in=w478, "Visible"=w475) -> (error out=w474:errorcluster)  [unwired: 1 in, 1 out]
              n155 = property on="Value" class="DigNum (strict)"(error in=w474, "Visible"=w476) -> (error out=w477:errorcluster)  [unwired: 1 in, 1 out]
              n156 = property on="Value 1/2" class="Enum (strict)"(error in=w477, "Visible"=w471) -> (error out=w470:errorcluster)  [unwired: 1 in, 1 out]
              n157 = property on="VISA resource name" class="VISAName"() -> ("Value"=w497:refnum<visa-resource-name>)  [unwired: 2 in, 2 out]
              n158 = property on="read buffer" class="Str"(error in=w469) -> (error out=w490:errorcluster, "Text.Scroll Position"=w487:u32)  [unwired: 1 in, 1 out]
              n159 = Or(x="Set", y="Get") -> (x .or. y?=w481:bool)
              n160 = case shown="\"Get\"" w482 {
                tunnel: "Function" -> [w561 _ w676]
                tunnel: w497 -> [w565 _ w686]
                tunnel: w490 -> [w563 w673 w674]
                tunnel: "Value" -> [_ _ w685]
                tunnel: "Value 1/2" -> [_ _ w683]
                tunnel: "Index" -> [w562 _ w680]
                tunnel: [w564 w673 w678] -> w489
                tunnel: [w559 w672 w677] -> w494
                tunnel: w481 -> [w558 _ w675]
                tunnel: w470 -> [_ _ _]
                frame "Get" {
                  n161 = disable-structure shown="Enabled" {
                    disable-tunnel: w563 -> [w568 _]
                    disable-tunnel: [w566 _] -> w560
                    frame Disabled {
                      w569 = TRUE ("Visible")
                      n162 = property on="Value" class="DigNum (strict)"(error in=w568, "Visible"=w569) -> (error out=w567:errorcluster)  [unwired: 1 in, 1 out]
                      n163 = property on="Value 1/2" class="Enum (strict)"(error in=w567, "Visible"=w569) -> (error out=w566:errorcluster)  [unwired: 1 in, 1 out]
                    }
                    frame Enabled {
                    }
                  }
                  n164 = case shown="True" w558 {
                    tunnel: w565 -> [_ w581]
                    tunnel: [w570 w577] -> w564
                    tunnel: w562 -> [_ w580]
                    tunnel: w561 -> [_ w579]
                    tunnel: w560 -> [w570 w578]
                    tunnel: [w571 w575] -> w559
                    frame False {
                      n165 = property on="read buffer" class="Str"() -> ("Value"=w571:string)  [unwired: 2 in, 2 out]
                    }
                    frame True {
                      w573 = FALSE ("Serial Send")
                      n166 = case shown="\"Serial Number\"" w579 {
                        tunnel: w581 -> [w585 w605 w624 w637 w647 w661 _]
                        tunnel: w578 -> [w584 w597 w615 w633 w646 w660 w670]
                        tunnel: [w588 w606 w625 w638 w651 w662 w670] -> w577
                        tunnel: [w587 w607 w623 w639 w652 w658 "Cannot perform operation.\n" ("read buffer")] -> w576
                        tunnel: w580 -> [_ w600 w616 _ _ _ _]
                        frame "Serial Number" {
                          n167 = disable-structure shown="Enabled" {
                            disable-tunnel: w584 -> [w592 w594]
                            disable-tunnel: [w591 w594] -> w583
                            frame Disabled {
                              n168 = property on="Index" class="Ring (strict)"(error in=w592, "DisabledEnum"=T11."Disabled and Grayed Out" ("Disabled")) -> (error out=w591:errorcluster)  [unwired: 1 in, 1 out]
                            }
                            frame Enabled {
                            }
                          }
                          n169 = Concatenate Strings("SN" ("string"), "\r\n" ("write buffer")) -> (w586:string)
                          n170 = call "Serial.vi"("error in (no error)"=w583, "Clear Log"=FALSE, "write buffer"=w586, "VISA resource name"=w585) -> ("error out"=w588:errorcluster, "read buffer"=w587:string)  [unwired: 6 in]
                        }
                        frame "Temperature" {
                          n171 = disable-structure shown="Enabled" {
                            disable-tunnel: w597 -> [w610 w612]
                            disable-tunnel: [w609 w612] -> w596
                            frame Disabled {
                              n172 = property on="Index" class="Ring (strict)"(error in=w610, "DisabledEnum"=T11."Enabled" ("Disabled"), "Visible"=TRUE) -> (error out=w609:errorcluster)  [unwired: 1 in, 1 out]
                            }
                            frame Enabled {
                            }
                          }
                          n173 = Number To Decimal String(number=w600) -> (decimal integer string=w599:string)  [unwired: 1 in]
                          n174 = Concatenate Strings("TA" ("string"), "[", w599, "]", "\r\n" ("write buffer")) -> (w601:string)
                          n175 = call "Serial.vi"("error in (no error)"=w596, "Clear Log"=FALSE, "write buffer"=w601, "VISA resource name"=w605) -> ("error out"=w606:errorcluster, "read buffer"=w607:string)  [unwired: 6 in]
                        }
                        frame "Unit Adress" {
                          n176 = disable-structure shown="Enabled" {
                            disable-tunnel: w615 -> [w628 w630]
                            disable-tunnel: [w627 w630] -> w614
                            frame Disabled {
                              n177 = property on="Index" class="Ring (strict)"(error in=w628, "DisabledEnum"=T11."Enabled" ("Disabled"), "Visible"=TRUE) -> (error out=w627:errorcluster)  [unwired: 1 in, 1 out]
                            }
                            frame Enabled {
                            }
                          }
                          n178 = Number To Decimal String(number=w616) -> (decimal integer string=w622:string)  [unwired: 1 in]
                          n179 = Concatenate Strings("UA" ("string"), "[", w622, "]", "\r\n" ("write buffer")) -> (w617:string)
                          n180 = call "Serial.vi"("error in (no error)"=w614, "Clear Log"=FALSE, "write buffer"=w617, "VISA resource name"=w624) -> ("error out"=w625:errorcluster, "read buffer"=w623:string)  [unwired: 6 in]
                        }
                        frame "Calibration" {
                          n181 = disable-structure shown="Enabled" {
                            disable-tunnel: w633 -> [w641 w643]
                            disable-tunnel: [w640 w643] -> w632
                            frame Disabled {
                              n182 = property on="Index" class="Ring (strict)"(error in=w641, "DisabledEnum"=T11."Disabled and Grayed Out" ("Disabled")) -> (error out=w640:errorcluster)  [unwired: 1 in, 1 out]
                            }
                            frame Enabled {
                            }
                          }
                          n183 = Concatenate Strings("CC" ("string"), "\r\n" ("write buffer")) -> (w635:string)
                          n184 = call "Serial.vi"("error in (no error)"=w632, "Clear Log"=FALSE, "write buffer"=w635, "VISA resource name"=w637) -> ("error out"=w638:errorcluster, "read buffer"=w639:string)  [unwired: 6 in]
                        }
                        frame "Velocity" {
                          n185 = disable-structure shown="Enabled" {
                            disable-tunnel: w646 -> [w654 w656]
                            disable-tunnel: [w653 w656] -> w645
                            frame Disabled {
                              n186 = property on="Index" class="Ring (strict)"(error in=w654, "DisabledEnum"=T11."Disabled and Grayed Out" ("Disabled")) -> (error out=w653:errorcluster)  [unwired: 1 in, 1 out]
                            }
                            frame Enabled {
                            }
                          }
                          n187 = Concatenate Strings("VC" ("string"), "\r\n" ("write buffer")) -> (w648:string)
                          n188 = call "Serial.vi"("error in (no error)"=w645, "Clear Log"=FALSE, "write buffer"=w648, "VISA resource name"=w647) -> ("error out"=w651:errorcluster, "read buffer"=w652:string)  [unwired: 6 in]
                        }
                        frame "Version" {
                          n189 = disable-structure shown="Enabled" {
                            disable-tunnel: w660 -> [w667 w669]
                            disable-tunnel: [w666 w669] -> w659
                            frame Disabled {
                              n190 = property on="Index" class="Ring (strict)"(error in=w667, "DisabledEnum"=T11."Disabled and Grayed Out" ("Disabled")) -> (error out=w666:errorcluster)  [unwired: 1 in, 1 out]
                            }
                            frame Enabled {
                            }
                          }
                          n191 = Concatenate Strings("VR" ("string"), "\r\n" ("write buffer")) -> (w663:string)
                          n192 = call "Serial.vi"("error in (no error)"=w659, "Clear Log"=FALSE, "write buffer"=w663, "VISA resource name"=w661) -> ("error out"=w662:errorcluster, "read buffer"=w658:string)  [unwired: 6 in]
                        }
                        frame Default {
                        }
                      }
                      n193 = property on="Serial Send" class="Bool (strict)"(error in=w577, "Value"=w573) -> (error out=w572:errorcluster)  [unwired: 1 in, 1 out]
                      n194 = property on="read buffer" class="Str"() -> ("Value"=w574:string)  [unwired: 2 in, 2 out]
                      n195 = Concatenate Strings(w574, w576) -> (w575:string)
                      n196 = property on="Get" class="Bool (strict)"(error in=w572, "Value"=w573) -> ()  [unwired: 1 in, 2 out]
                    }
                  }
                }
                frame Default {
                  n197 = property on="read buffer" class="Str"() -> ("Value"=w672:string)  [unwired: 2 in, 2 out]
                }
                frame "Set" {
                  n198 = To Unsigned Long Integer(number=w685) -> (unsigned 32bit integer=w681:u32)
                  n199 = Number To Decimal String(number=w680) -> (decimal integer string=w679:string)  [unwired: 1 in]
                  n200 = Number To Decimal String(number=w683) -> (decimal integer string=w682:string)  [unwired: 1 in]
                  n201 = Number To Decimal String(number=w681) -> (decimal integer string=w684:string)  [unwired: 1 in]
                  n202 = case shown="True" w675 {
                    tunnel: w686 -> [_ w703]
                    tunnel: w684 -> [_ w702]
                    tunnel: w682 -> [_ w701]
                    tunnel: w681 -> [_ w700]
                    tunnel: w679 -> [_ w699]
                    tunnel: [w687 w690] -> w678
                    tunnel: [w688 w698] -> w677
                    tunnel: w676 -> [_ w696]
                    tunnel: w674 -> [w687 w695]
                    frame False {
                      n203 = property on="read buffer" class="Str"() -> ("Value"=w688:string)  [unwired: 2 in, 2 out]
                    }
                    frame True {
                      w689 = TRUE ("Value (Signaling)")
                      w692 = FALSE ("Serial Send")
                      n204 = flat-sequence {
                        tunnel: [w707] -> w705
                        tunnel: w695 -> [w707]
                        frame #0 {
                          n205 = Wait (ms)(milliseconds to wait=u32 50) -> ()  [unwired: 1 out]
                        }
                      }
                      n206 = case shown="\"Velocity\"" w696 {
                        tunnel: [w711 w718 w728 w737 w756 "EP=1\r\n" ("write buffer") "Cannot perform operation.\n" ("read buffer")] -> w697
                        tunnel: w705 -> [w710 w717 w727 w742 w747 w759 w761]
                        tunnel: [w710 w717 w727 w742 w744 w759 w761] -> w704
                        tunnel: w702 -> [w712 w719 w733 _ _ _ _]
                        tunnel: w701 -> [_ _ _ w738 _ _ _]
                        tunnel: w700 -> [_ _ _ _ w748 _ _]
                        tunnel: w699 -> [_ w720 w731 _ _ _ _]
                        tunnel: "EP=1\r\n" ("string") -> [w709 w716 w726 w736 w743 _ _]
                        frame "Serial Number" {
                          n207 = Concatenate Strings(w709, "SN" ("write buffer"), "=" ("string"), w712, "\r\n" ("write buffer")) -> (w711:string)
                        }
                        frame "Temperature" {
                          n208 = Concatenate Strings(w716, "TA" ("string"), "[", w720, "]", "=" ("string"), w719, "\r\n" ("write buffer")) -> (w718:string)
                        }
                        frame "Unit Adress" {
                          n209 = Concatenate Strings(w726, "UA" ("string"), "[", w731, "]", "=" ("string"), w733, "\r\n" ("write buffer")) -> (w728:string)
                        }
                        frame "Calibration" {
                          n210 = Concatenate Strings(w736, "CC" ("string"), "=" ("string"), w738, "\r\n" ("write buffer")) -> (w737:string)
                        }
                        frame "Velocity" {
                          n211 = In Range and Coerce(upper limit=u16 18001, x=w748, lower limit=u16 0) -> (coerced(x)=w754:u32, In Range?=w752:bool)
                          n212 = Not(x=w752) -> (.not. x?=w753:bool)
                          n213 = Select(t=w754, s=w752, f=u16 0) -> (s? t:f=w746:u32)
                          n214 = Number To Decimal String(number=w746) -> (decimal integer string=w745:string)  [unwired: 1 in]
                          n215 = Concatenate Strings(w743, "VC" ("write buffer"), "=" ("string"), w745, "\r\n" ("write buffer")) -> (w756:string)
                          n216 = call "Display Message to User2"("error in (no error)"=w747, "Enable"=w753) -> ("error out"=w744:errorcluster)  [unwired: 8 in, 1 out]
                        }
                        frame "Enable Conf. EP=1" {
                        }
                        frame Default {
                        }
                      }
                      n217 = property on="read buffer" class="Str"() -> ("Value"=w694:string)  [unwired: 2 in, 2 out]
                      n218 = VISA Write(VISA resource name=w703, write buffer=w697, error in (no error)=w704) -> (error out=w706:errorcluster)  [unwired: 2 out]
                      n219 = Concatenate Strings(w694, w697) -> (w698:string)
                      n220 = property on="Serial Send" class="Bool (strict)"("Value"=w692) -> ()  [unwired: 2 in, 2 out]
                      n221 = flat-sequence {
                        tunnel: w706 -> [w763]
                        tunnel: [w763] -> w691
                        frame #0 {
                          n222 = Wait (ms)(milliseconds to wait=u32 50) -> ()  [unwired: 1 out]
                        }
                      }
                      n223 = property on="Get" class="Bool (strict)"(error in=w691, "Val(Sgnl)"=w689, "Value"=w689) -> (error out=w690:errorcluster)  [unwired: 1 in, 1 out]
                      n224 = property on="Set" class="Bool (strict)"("Value"=w692) -> ()  [unwired: 2 in, 2 out]
                    }
                  }
                }
              }
              "read buffer" <- w494
              n225 = Add(x=u32 5, y=w487) -> (x+y=w486:u32)
              n226 = property on="read buffer" class="Str"(error in=w489, "Text.Scroll Position"=w486) -> (error out=w488:errorcluster)  [unwired: 1 in, 1 out]
            }
            event "Set Param.": Value Change {
              n227 = event-data() -> ()  [unwired: 1 in, 6 out]
              n228 = property on="Serial Status" class="Bool (strict)"(error in=w769) -> (error out=w768:errorcluster, "Value"=w773:bool)  [unwired: 1 in, 1 out]
              n229 = case shown="True" w773 {
                tunnel: w768 -> [w785 w798]
                tunnel: [w784 w794] -> w771
                frame False {
                  n230 = call "Display Message to User4"("error in (no error)"=w785) -> ("error out"=w784:errorcluster)  [unwired: 9 in, 1 out]
                }
                frame True {
                  w787 = FALSE ("Visible")
                  n231 = property on="Speed control" class="Bool (strict)"(error in=w798, "Visible"=FALSE) -> (error out=w797:errorcluster)  [unwired: 1 in, 1 out]
                  n232 = case shown="47" "Param to Set" {
                    tunnel: [w851 w855 w859] -> w813
                    tunnel: w797 -> [w850 w854 w858]
                    tunnel: [w850 w854 w858] -> w801
                    frame 95, Default {
                      n233 = call <vilib>:"Application Directory.vi"() -> ("Application Directory"=w853:path)
                      n234 = Build Path(base path=w853, name or relative path="data\\Marvin_EBAY_params_RRPAR000017_95_v0.2.txt") -> (appended path=w851:path)
                    }
                    frame 63 {
                      n235 = call <vilib>:"Application Directory.vi"() -> ("Application Directory"=w857:path)
                      n236 = Build Path(base path=w857, name or relative path="data\\Marvin_AHU_params_RRPAR000016_63_v0.2.txt") -> (appended path=w855:path)
                    }
                    frame 47 {
                      n237 = call <vilib>:"Application Directory.vi"() -> ("Application Directory"=w861:path)
                      n238 = Build Path(base path=w861, name or relative path="data\\Marvin_AHU_params_RRPAR000015_47_v0.2.txt") -> (appended path=w859:path)
                    }
                  }
                  n239 = property on="read buffer" class="Str"(error in=w801, "Visible"=TRUE) -> (error out=w789:errorcluster)  [unwired: 1 in, 1 out]
                  n240 = property on="CAN Data" class="Arr (strict)"(error in=w789, "Visible"=w787) -> (error out=w788:errorcluster)  [unwired: 1 in, 1 out]
                  n241 = property on="PlayPause Data Array" class="Bool (strict)"("Visible"=w787) -> ()  [unwired: 2 in, 2 out]
                  n242 = property on="Clear Data Array" class="Bool (strict)"("Visible"=w787) -> ()  [unwired: 2 in, 2 out]
                  n243 = property on="Horizontal Progress Bar" class="Slide (strict)"(error in=w788, "Visible"=TRUE, "Value"=u8 0 ("Horizontal Progress Bar")) -> (error out=w796:errorcluster)  [unwired: 1 in, 1 out]
                  n244 = call <vilib>:"Read Characters From File.vi"("file path (dialog if empty)"=w813) -> ("character string"=w814:string)  [unwired: 5 in, 3 out]
                  n245 = while {
                    shift-right: [w842] -> _
                    shift-left: w814 -> [w843]
                    shift-right: [w838] -> w799
                    shift-left: string[] [] -> [w839]
                    tunnel: w796 -> [w831]
                    tunnel: [w831] -> w811
                    stop <- w844 stop-if-true
                    n246 = Match Pattern(string=w843, regular expression="\r\n") -> (before substring=w840:string, after substring=w842:string, offset past match=w841:i32)  [unwired: 1 in, 1 out]
                    n247 = call <vilib>:"Trim Whitespace.vi"("string"=w840) -> ("trimmed string"=w837:string)  [unwired: 1 in]
                    n248 = Equal?(x=w841, y=-1) -> (x = y?=w844:bool)
                    n249 = To Upper Case(1:w837) -> (0:w835:string)
                    n250 = String Length(string=w835) -> (length=w834:i32)
                    n251 = Greater?(x=w834, y=3) -> (0:w832:bool)
                    n252 = case shown="True" w832 {
                      tunnel: w839 -> [w846 w849]
                      tunnel: [w846 w848] -> w838
                      tunnel: w835 -> [_ w847]
                      frame False {
                      }
                      frame True {
                        n253 = Build Array (concatenate)(w849, w847) -> (w848:string[])
                      }
                    }
                  }
                  n254 = property on="VISA resource name" class="VISAName"(error in=w811) -> (error out=w804:errorcluster, "Value"=w793:refnum<visa-resource-name>)  [unwired: 1 in, 1 out]
                  n255 = Build Array (concatenate)(w799, string[] ["MT", "VR", "SN"] ("array")) -> (w808:string[])
                  n256 = Array Size(array=w808) -> (size(s)=w800:i32)
                  n257 = Bundle By Name(cluster=T12 {"Minimum"=0.0, "Maximum"=0.0, "Increment"=0.0} ("Data Entry Limits"), "Minimum"=0.0, "Maximum"=w800) -> (w806:T12)
                  n258 = property on="Horizontal Progress Bar" class="Slide (strict)"(error in=w804, "Data Range"=w806) -> (error out=w792:errorcluster)  [unwired: 1 in, 1 out]
                  n259 = property on="read buffer" class="Str"(error in=w792) -> (error out=w791:errorcluster, "Text.Scroll Position"=w790:u32)  [unwired: 1 in, 1 out]
                  n260 = for {
                    tunnel: w808 -> [w822] mode=indexing
                    tunnel: w793 -> [w828]
                    tunnel: w791 -> [w827]
                    tunnel: [w819] -> w795
                    tunnel: w790 -> [w818]
                    i -> [w817]
                    n261 = Concatenate Strings(w822, "\r\n" ("string")) -> (w820:string)
                    n262 = VISA Write(VISA resource name=w828, write buffer=w820, error in (no error)=w827) -> (error out=w826:errorcluster)  [unwired: 2 out]
                    n263 = flat-sequence {
                      tunnel: w826 -> [w829]
                      tunnel: [w829] -> w819
                      frame #0 {
                        n264 = Wait (ms)(milliseconds to wait=u32 50) -> ()  [unwired: 1 out]
                      }
                    }
                    n265 = Add(x=w818, y=w817) -> (x+y=w816:u32)
                    n266 = feedback #1("") -> (w824:string)
                    n267 = Concatenate Strings(w824, w820) -> (w825:string)
                    n268 = feedback-in #1(w825) -> ()
                    n269 = property on="read buffer" class="Str"("Value"=w825, "Text.Scroll Position"=w816) -> ()  [unwired: 2 in, 2 out]
                    "Horizontal Progress Bar" <- w817
                  }
                  n270 = VISA Flush I/O Buffer(VISA resource name=w793, error in (no error)=w795) -> (error out=w794:errorcluster)  [unwired: 1 in, 1 out]
                }
              }
              n271 = property on="Serial Monitor" class="Bool (strict)"(error in=w771) -> (error out=w770:errorcluster, "Value"=w772:bool)  [unwired: 1 in, 1 out]
              n272 = case shown="False" w772 {
                tunnel: w770 -> [w782 w783]
                tunnel: [w779 w783] -> w766
                frame False {
                  w778 = TRUE ("Visible")
                  n273 = property on="PlayPause Data Array" class="Bool (strict)"("Visible"=w778) -> ()  [unwired: 2 in, 2 out]
                  n274 = property on="read buffer" class="Str"(error in=w782, "Visible"=FALSE) -> (error out=w780:errorcluster)  [unwired: 1 in, 1 out]
                  n275 = property on="Clear Data Array" class="Bool (strict)"("Visible"=w778) -> ()  [unwired: 2 in, 2 out]
                  n276 = property on="CAN Data" class="Arr (strict)"(error in=w780, "Visible"=w778) -> (error out=w779:errorcluster)  [unwired: 1 in, 1 out]
                }
                frame True {
                }
              }
              n277 = call "Display Message to User5"("error in (no error)"=w766) -> ("error out"=w765:errorcluster)  [unwired: 9 in, 1 out]
            }
            event "Help Button": Value Change {
              n278 = event-data() -> ()  [unwired: 1 in, 6 out]
              n279 = control-ref of="This VI"() -> (w870:refnum<vi>)
              n280 = property class="VI"(reference=w870, error in=w868, "FP:Transparency"=u8 25 ("Front Panel Window:Transparency")) -> (reference out=w864:refnum<vi>, error out=w867:errorcluster)
              n281 = vi-ref "Help.vi"() -> (w874:refnum<vi>)
              n282 = invoke class="VI" method="FP.Open"(reference=w874, error in=w867, "Activate"=TRUE ("Activate?"), "State"=T13."Standard") -> (error out=w873:errorcluster)  [unwired: 1 in, 4 out]
              n283 = call "Help.vi"("error in"=w873, "TesterSWVersion"="1.7") -> ("error out"=w866:errorcluster)  [unwired: 6 in]
              n284 = property class="VI"(reference=w864, error in=w866, "FP:Transparency"=u8 0 ("Front Panel Window:Transparency")) -> (error out=w865:errorcluster)  [unwired: 1 out]
            }
            event "Can Send": Value Change {
              w902 = u8 0 items=["STATUS"=128, "EXTENDED"=2, "RTR"=1, "DATA MSG"=0] ("MSGTYPE")
              w907 = u8 1 items=["Standart flag", "Extern flag"] ("Format")
              w906 = u8 0 items=["Data flag", "Remote flag"] ("Type")
              # "Send"
              n285 = event-data() -> ()  [unwired: 1 in, 6 out]
              n286 = disable-structure shown="Disabled" {
                disable-tunnel: "Motor Phase Current" -> [w920 _]
                frame Disabled {
                  w921 = u16 40 ("lower limit")
                  n287 = In Range and Coerce(upper limit=u16 100, x=w920, lower limit=w921) -> (coerced(x)=w923:u16, In Range?=w925:bool)
                  n288 = Not(x=w925) -> (.not. x?=w924:bool)
                  n289 = call "Display Message to User6"("Enable"=w924) -> ()  [unwired: 9 in, 2 out]
                  n290 = Select(t=w923, s=w925, f=w921) -> ()  [unwired: 1 out]
                }
                frame Enabled {
                }
              }
              n291 = In Range and Coerce(upper limit=u16 18001, x="Motor Speed RPM", lower limit=u16 0) -> (coerced(x)=w889:u16, In Range?=w887:bool)
              n292 = Not(x=w887) -> (.not. x?=w888:bool)
              n293 = call "Display Message to User"("Enable"=w888) -> ()  [unwired: 9 in, 2 out]
              n294 = Select(t=w889, s=w887, f=u16 0) -> (s? t:f=w891:u16)
              n295 = property on="UUT" class="DigNum (strict)"() -> ("Value"=w885:u8)  [unwired: 2 in, 2 out]
              n296 = Split Number(x=w891) -> (hi(x)=w894:u8, lo(x)=w895:u8)
              n297 = case shown="79" w885 {
                tunnel: [u32 417357607 u32 417353511 u32 417349415 u32 417345319] -> w886
                frame 95, Default {
                }
                frame 79 {
                }
                frame 63 {
                }
                frame 47 {
                }
              }
              n298 = case shown="79" w885 {
                tunnel: [w932 w941 w954 w968] -> w900
                tunnel: w895 -> [w931 w940 w953 w967]
                tunnel: w894 -> [w930 w939 w952 w966]
                tunnel: "Motor Speed RPM" -> [w927 w936 _ _]
                tunnel: "Speed control" -> [_ _ w945 w959]
                tunnel: "Motor Over Temp" -> [_ _ w944 w958]
                tunnel: "Motor Phase Current" -> [_ _ _ w955]
                frame 47, Default {
                  w929 = u8 0 ("element")
                  n299 = case shown="1, Default" w927 {
                    tunnel: [u8 1 ("element") u8 0 ("element")] -> w926
                    frame 1, Default {
                    }
                    frame 0 {
                    }
                  }
                  n300 = Build Array(u8 1 ("element"), w931, w930, w926, w929, w929, w929, w929) -> (w932:u8[])
                }
                frame 63 {
                  w937 = u8 0 ("element")
                  n301 = case shown="1, Default" w936 {
                    tunnel: [u8 1 ("element") u8 0 ("element")] -> w935
                    frame 1, Default {
                    }
                    frame 0 {
                    }
                  }
                  n302 = Build Array(u8 1 ("element"), w940, w939, w935, w937, w937, w937, w937) -> (w941:u8[])
                }
                frame 95 {
                  w950 = u8 0 ("element")
                  n303 = Boolean To (0,1)(Boolean=w945) -> (0, 1=w948:i16)
                  n304 = Boolean To (0,1)(Boolean=w944) -> (0, 1=w949:i16)
                  n305 = To Unsigned Byte Integer(number=w948) -> (unsigned 8bit integer=w947:u8)
                  n306 = To Unsigned Byte Integer(number=w949) -> (unsigned 8bit integer=w946:u8)
                  n307 = Build Array(u8 1 ("element"), w953, w952, w947, w946, w950, w950, w950) -> (w954:u8[])
                }
                frame 79 {
                  n308 = Split Number(x=w955) -> (hi(x)=w956:u8, lo(x)=w957:u8)
                  n309 = Boolean To (0,1)(Boolean=w959) -> (0, 1=w962:i16)
                  n310 = Boolean To (0,1)(Boolean=w958) -> (0, 1=w963:i16)
                  n311 = To Unsigned Byte Integer(number=w962) -> (unsigned 8bit integer=w961:u8)
                  n312 = To Unsigned Byte Integer(number=w963) -> (unsigned 8bit integer=w960:u8)
                  n313 = Build Array(u8 1 ("element"), w967, w966, w961, w960, w957, w956, u8 0 ("element")) -> (w968:u8[])
                }
              }
              n314 = Array Size(array=w900) -> (size(s)=w905:i32)
              n315 = call "Array Data to Single Num in Hex.vi"("aDATA"=w900) -> ("Numeric"=→"Data Send":u64)  [unwired: 10 in]
              n316 = To Unsigned Byte Integer(number=w905) -> (unsigned 8bit integer=w903:u8)
              n317 = call "CANAnalData.vi"("ID"=w886, "Data"=w900, "Config"=w898) -> ()  [unwired: 4 in, 5 out]
              n318 = Bundle By Name(cluster=T10 {"ID"=0, "MSGTYPE"=0, "LEN"=0, "aDATA"=[]} ("MsgTX 2"), "ID"=w886, "MSGTYPE"=w902, "LEN"=w903, "aDATA"=w900) -> (w901:T10)
              n319 = Unbundle By Name(w901) -> ("ID"=w915:u32, "LEN"=w916:u8, "aDATA"=w917:u8[])  [unwired: 1 out]
              n320 = property class="Clust (strict)"(reference=w898) -> ("Value"=w914:T8)  [unwired: 1 in, 2 out]
              n321 = Bundle By Name(cluster=T14 {"ID"=0, "TimeStamp"=0, "TimeFlag"=0, "SendType"=0, "RemoteFlag"=0, "ExternFlag"=0, "DataLen"=0, "Data"=[], "Reserved"=[]} ("Send"), "ID"=w915, "RemoteFlag"=w906, "ExternFlag"=w907, "DataLen"=w916, "Data"=w917) -> (w912:T14)
              n322 = Unbundle By Name(w914) -> ("DevType"=w908:T2, "DevIndex"=w909:u32, "CanIndex"=w910:T3)
              n323 = Build Array(w912) -> (w911:T14[])
              n324 = call "VCI_Transmit.vi"("Buffer"=w911, "CANIndex"=w910, "DevIndex"=w909, "DevType"=w908) -> ()  [unwired: 1 in, 7 out]
            }
            event "Graph Button": Value Change {
              w974 = FALSE ("Visible")
              w976 = FALSE ("Visible")
              n325 = event-data() -> ()  [unwired: 1 in, 6 out]
              n326 = Not(x="Graph Button") -> (.not. x?=w977:bool)
              n327 = property on="PlayPause Data Array" class="Bool (strict)"("Visible"=w977) -> ()  [unwired: 2 in, 2 out]
              n328 = property on="CAN Data" class="Arr (strict)"(error in=w978, "Visible"=w977) -> (error out=w979:errorcluster)  [unwired: 1 in, 1 out]
              n329 = property on="Clear Data Array" class="Bool (strict)"("Visible"=w977) -> ()  [unwired: 2 in, 2 out]
              n330 = property on="Waveform Chart" class="WFChart (strict)"(error in=w979, "Visible"="Graph Button") -> (error out=w981:errorcluster)  [unwired: 1 in, 1 out]
              n331 = property on="Serial Monitor" class="Bool (strict)"(error in=w981) -> (error out=w994:errorcluster, "Value"=w995:bool)  [unwired: 1 in, 1 out]
              n332 = case shown="True" w995 {
                tunnel: w994 -> [w1002 w1007]
                tunnel: [w1000 w1004] -> w984
                frame False {
                  n333 = property on="read buffer" class="Str"(error in=w1002, "Visible"=FALSE) -> (error out=w1000:errorcluster)  [unwired: 1 in, 1 out]
                }
                frame True {
                  w1003 = FALSE ("Visible")
                  n334 = property on="PlayPause Data Array" class="Bool (strict)"("Visible"=w1003) -> ()  [unwired: 2 in, 2 out]
                  n335 = property on="read buffer" class="Str"(error in=w1007, "Visible"=TRUE) -> (error out=w1005:errorcluster)  [unwired: 1 in, 1 out]
                  n336 = property on="Clear Data Array" class="Bool (strict)"("Visible"=w1003) -> ()  [unwired: 2 in, 2 out]
                  n337 = property on="CAN Data" class="Arr (strict)"(error in=w1005, "Visible"=w1003) -> (error out=w1004:errorcluster)  [unwired: 1 in, 1 out]
                }
              }
              n338 = property on="Serial Monitor" class="Bool (strict)"(error in=w984, "Value"=FALSE ("Serial Monitor")) -> (error out=w982:errorcluster)  [unwired: 1 in, 1 out]
              n339 = property on="Index" class="Ring (strict)"(error in=w982, "Visible"=w976) -> (error out=w991:errorcluster)  [unwired: 1 in, 1 out]
              n340 = property on="Value 1/2" class="Enum (strict)"(error in=w991, "Visible"=w976) -> (error out=w990:errorcluster)  [unwired: 1 in, 1 out]
              n341 = property on="Value" class="DigNum (strict)"(error in=w990, "Visible"=w976) -> (error out=w989:errorcluster)  [unwired: 1 in, 1 out]
              n342 = property on="SetGet" class="Enum (strict)"(error in=w989, "Visible"=w976) -> (error out=w973:errorcluster)  [unwired: 1 in, 1 out]
              n343 = property on="Set" class="Bool (strict)"(error in=w973, "Visible"=w974) -> (error out=w975:errorcluster)  [unwired: 1 in, 1 out]
              n344 = property on="Get" class="Bool (strict)"(error in=w975, "Visible"=w974) -> ()  [unwired: 1 in, 2 out]
              n345 = property on="Serial Send" class="Bool (strict)"(error in=w973, "Visible"=w976) -> (error out=w987:errorcluster)  [unwired: 1 in, 1 out]
              n346 = property on="Clear Monitor" class="Bool"(error in=w987, "Visible"=w976) -> (error out=w986:errorcluster)  [unwired: 1 in, 1 out]
              n347 = property on="Function" class="Enum (strict)"(error in=w986, "Visible"=w976) -> (error out=w988:errorcluster)  [unwired: 1 in, 1 out]
              n348 = property on="Index" class="Ring (strict)"(error in=w988, "Visible"=w976) -> (error out=w992:errorcluster)  [unwired: 1 in, 1 out]
              n349 = property on="read buffer" class="Str"(error in=w992, "Visible"=w976) -> (error out=w985:errorcluster)  [unwired: 1 in, 1 out]
            }
            event "Serial Com": Value Change {
              n350 = event-data() -> ()  [unwired: 1 in, 6 out]
              n351 = property on="Serial Com" class="Bool"(error in=w1012, "Visible"=FALSE) -> (error out=w1011:errorcluster)  [unwired: 1 in, 1 out]
              n352 = property on="VISA resource name" class="VISAName"(error in=w1011, "Visible"=TRUE) -> (error out=w1009:errorcluster)  [unwired: 1 in, 1 out]
            }
            event "VISA resource name": Value Change {
              n353 = event-data() -> ()  [unwired: 1 in, 1 out]
              n354 = control-ref of="This VI"() -> (w1018:refnum<vi>)
              n355 = call "Serial InitMarvin.vi"("error in (no error)"=w1027, "VI reference (current VI)"=w1018, "VISA Refnum in"="VISA resource name") -> ("error out"=w1036:errorcluster, "Boolean"=w1024:bool)  [unwired: 7 in]
              n356 = property on="Serial Status" class="Bool (strict)"(error in=w1036, "Value"=w1024) -> (error out=w1030:errorcluster)  [unwired: 1 in, 1 out]
              n357 = property on="VISA resource name" class="VISAName"(error in=w1030, "Visible"=FALSE) -> (error out=w1029:errorcluster)  [unwired: 1 in, 1 out]
              n358 = property on="Serial Com" class="Bool"(error in=w1029, "Visible"=TRUE) -> (error out=w1022:errorcluster)  [unwired: 1 in, 1 out]
              n359 = call "Serial.vi"("error in (no error)"=w1022, "Clear Log"=TRUE, "VISA resource name"="VISA resource name") -> ("error out"=w1020:errorcluster)  [unwired: 7 in, 1 out]
              n360 = call <vilib>:"Clear Errors.vi"("error in (no error)"=w1020) -> ("error out"=w1026:errorcluster)  [unwired: 5 in, 1 out]
              n361 = case shown="True" w1024 {
                tunnel: w1026 -> [w1037 w1040]
                tunnel: [w1037 w1039] -> w1025
                tunnel: "VISA resource name" -> [_ w1038]
                frame False {
                }
                frame True {
                  n362 = VISA Flush I/O Buffer(VISA resource name=w1038, error in (no error)=w1040) -> (error out=w1039:errorcluster)  [unwired: 1 in, 1 out]
                }
              }
            }
            event "Stop": Value Change {
              n363 = event-data() -> ()  [unwired: 1 in, 6 out]
              n364 = Flush Queue(queue=w1046, error in (no error)=w1045) -> (queue out=w1044:refnum<queue>, error out=w1043:errorcluster)  [unwired: 1 out]
              n365 = Release Queue(queue=w1044, error in (no error)=w1043) -> (error out=w1042:errorcluster)  [unwired: 1 in, 2 out]
            }
            event "Refresh Button", "Graph Plot": Value Change {
              n366 = event-data() -> ("CtlRef"=w1053:refnum<vi>)  [unwired: 1 in, 5 out]
              n367 = property class="Bool"(reference=w1053) -> ("Label.Text"=w1052:string)  [unwired: 1 in, 2 out]
              n368 = case shown="\"Graph Plot\"" w1052 {
                tunnel: w1057 -> [w1062 w1066 w1071]
                tunnel: w1056 -> [_ _ w1070]
                tunnel: [w1063 w1066 w1069] -> w1055
                tunnel: [FALSE ("Stop") FALSE ("Stop") TRUE ("Stop")] -> w1051
                tunnel: [enum16{"Stop", "MainProgram", "Initialize"}."MainProgram" enum16{"Stop", "MainProgram", "Initialize"}."MainProgram" enum16{"Stop", "MainProgram", "Initialize"}."Initialize"] -> w1050
                frame "Graph Plot" {
                  n369 = property on="Waveform Chart" class="WFChart (strict)"(error in=w1062, "History Data"=dbl[] [] ("Waveform Chart")) -> (error out=w1063:errorcluster)  [unwired: 1 in, 1 out]
                }
                frame Default {
                }
                frame "Refresh Button" {
                  n370 = Release Queue(queue=w1070, error in (no error)=w1071) -> (error out=w1069:errorcluster)  [unwired: 1 in, 2 out]
                }
              }
            }
          }
          n371 = Unbundle By Name(w283) -> ("status"=w289:bool)
          n372 = Or(x=w289, y=w281) -> (x .or. y?=w288:bool)
        }
        n373 = while {
          shift-right: [w124] -> _
          shift-left: w101 -> [w125]
          shift-right: [w122] -> _
          shift-left: _ -> [w123]
          shift-right: [w118] -> _
          shift-left: w100 -> [w118]
          shift-right: [w107] -> w96
          shift-left: w97 -> [w110]
          shift-right: [w111] -> _
          shift-left: cluster{"Frame Data":u64, "Frame ID":u32}[] [] ("Array 3") -> [w113]
          stop <- w108 stop-if-true
          n374 = Dequeue Element(queue=w125, error in (no error)=w118) -> (queue out=w124:refnum<queue>, element=w119:T9, error out=w108:errorcluster)  [unwired: 1 in, 1 out]
          n375 = for {
            tunnel: [w267] -> w121 mode=indexing
            tunnel: w119 -> [w269] mode=indexing
            tunnel: [w268] -> w120 mode=indexing
            tunnel: [w266] -> w117 mode=indexing
            tunnel: [w265] -> w116 mode=indexing
            shift-right: [w265] -> _
            shift-left: _ -> [w264]
            n376 = Unbundle By Name(w269) -> ("ID"=w266:u32, "aDATA"=w268:u8[])
            n377 = call "Array Data to Single Num in Hex.vi"("aDATA"=w268) -> ("Numeric"=w267:u64)  [unwired: 10 in]
            n378 = case shown="Default" w266 {
              tunnel: w267 -> [_ w274]
              tunnel: w266 -> [_ w273]
              tunnel: [w270 w272] -> w265
              tunnel: w264 -> [w270 _]
              frame 0 {
              }
              frame Default {
                n379 = Bundle By Name(cluster=cluster{"Frame Data":u64, "Frame ID":u32} {"Frame Data"=0, "Frame ID"=0} ("Cluster"), "Frame ID"=w273, "Frame Data"=w274) -> (w272:cluster{"Frame Data":u64, "Frame ID":u32})
              }
            }
          }
          n380 = case shown="True" "PlayPause Data Array" {
            tunnel: w116 -> [w128 _]
            tunnel: w113 -> [w127 w129]
            tunnel: [w126 w129] -> w112
            frame False {
              n381 = Build Array (concatenate)(w128, w127) -> (w126:cluster{"Frame Data":u64, "Frame ID":u32}[])
            }
            frame True {
            }
          }
          n382 = Build Array (concatenate)(w121, w123) -> (w122:u64[][])
          "Array" <- w122
          n383 = Select(t=cluster{"Frame Data":u64, "Frame ID":u32}[] [], s="Clear Data Array", f=w112) -> (s? t:f=w111:cluster{"Frame Data":u64, "Frame ID":u32}[])
          "CAN Data" <- w111
          n384 = for {
            tunnel: w120 -> [w133] mode=indexing
            tunnel: w117 -> [w131] mode=indexing
            shift-right: [w130] -> w107
            shift-left: w110 -> [w132]
            n385 = case shown="417474367, 417474383, 417474399" w131 {
              tunnel: w133 -> [_ w163 w201 w259]
              tunnel: [w134 w136 w192 w231] -> w130
              tunnel: w132 -> [w134 w140 w192 w232]
              frame Default {
              }
              frame 417408831, 417408847, 417408863 {
                # "Frame ID\n0x18E1273F"
                n386 = Index Array(array=w163, index #1=0 ("index"), index #2=1 ("index"), index #3=2 ("index"), index #4=3 ("index"), index #5=4 ("index"), index #6=5 ("index"), index #7=6 ("index"), index #8=7 ("index")) -> (element #1=w147:u8, element #2=w149:u8, element #3=w150:u8, element #4=w154:u8, element #5=w157:u8, element #6=w161:u8, element #7=w162:u8, element #8=w160:u8)
                n387 = Join Numbers(hi=w162, lo=w161) -> ((hi.lo)=w181:u16)
                n388 = Join Numbers(hi=w150, lo=w149) -> ((hi.lo)=w151:u16)
                n389 = Number To Hexadecimal String(2:w181) -> (0:w180:string)  [unwired: 1 in]
                n390 = Number To Hexadecimal String(2:w160) -> (0:w174:string)  [unwired: 1 in]
                n391 = Number To Hexadecimal String(2:w147) -> (0:w148:string)  [unwired: 1 in]
                n392 = Number To Hexadecimal String(2:w151) -> (0:w152:string)  [unwired: 1 in]
                n393 = Number To Hexadecimal String(2:w154) -> (0:w155:string)  [unwired: 1 in]
                n394 = Number To Hexadecimal String(2:w157) -> (0:w158:string)  [unwired: 1 in]
                n395 = Hexadecimal String To Number(string=w148) -> (number=w145:u32)  [unwired: 2 in, 1 out]
                n396 = Hexadecimal String To Number(string=w152) -> (number=w153:u32)  [unwired: 2 in, 1 out]
                n397 = Hexadecimal String To Number(string=w155) -> (number=w156:u32)  [unwired: 2 in, 1 out]
                n398 = Hexadecimal String To Number(string=w158) -> (number=w159:u32)  [unwired: 2 in, 1 out]
                n399 = Hexadecimal String To Number(string=w174) -> (number=w173:u32)  [unwired: 2 in, 1 out]
                n400 = Hexadecimal String To Number(string=w180) -> (number=w179:u32)  [unwired: 2 in, 1 out]
                n401 = To Unsigned Word Integer(number=w145) -> (unsigned 16bit integer=→"ECS State":u16)
                n402 = To Double Precision Float(number=w153) -> (double precision float=w139:dbl)
                "Motor Speed RPM" <- w139
                n403 = To Double Precision Float(number=w179) -> (double precision float=w176:dbl)
                n404 = To Double Precision Float(number=w173) -> (double precision float=→"DC Current":dbl)
                n405 = To Double Precision Float(number=w156) -> (double precision float=w144:dbl)
                n406 = To Double Precision Float(number=w159) -> (double precision float=w142:dbl)
                n407 = To Double Precision Float(number=u32 10 ("y")) -> (double precision float=w177:dbl)
                n408 = Subtract(x=w142, y=50.0 ("x")) -> (x-y=→"Power transistor Heat sink Temp.":dbl)
                n409 = Subtract(x=w144, y=50.0 ("x")) -> (x-y=→"Motor Stator Temp.":dbl)
                n410 = Divide(x=w176, y=w177) -> (x/y=→"DC Voltage":dbl)
                n411 = case shown="False" "Graph Plot" {
                  tunnel: w140 -> [w184 w189]
                  tunnel: [w182 w189] -> w136
                  tunnel: w139 -> [w183 _]
                  frame False {
                    n412 = disable-structure shown="Disabled" {
                      disable-tunnel: w183 -> [w188 _]
                      frame Disabled {
                        n413 = call <vilib>:"Application Directory.vi"() -> ("Application Directory"=w186:path)
                        n414 = Build Path(base path=w186, name or relative path="RPM Log.lvm") -> (appended path=w187:path)
                        n415 = call "Write To Measurement File"("Signals"=w188, "Filename"=w187) -> ()  [unwired: 15 in, 3 out]
                      }
                      frame Enabled {
                      }
                    }
                    n416 = Build Array (concatenate)(w183, w184) -> (w182:dbl[])
                    "Waveform Chart" <- w183
                  }
                  frame True {
                  }
                }
              }
              frame 417539903, 417539919, 417539935 {
                # "Framde ID\n0x18E3273F"
                n417 = property on="UUT" class="DigNum (strict)"() -> ("Value"=w191:u8)  [unwired: 2 in, 2 out]
                n418 = Index Array(array=w201, index #1=0 ("index"), index #2=1 ("index")) -> (element #1=w199:u8, element #2=w194:u8)
                n419 = case shown="Default" w191 {
                  tunnel: [0 1 2] -> w190
                  frame Default {
                  }
                  frame 95 {
                  }
                  frame 79 {
                  }
                }
                n420 = Number To Boolean Array(number=w199) -> (Boolean array=w198:bool[])
                n421 = Number To Boolean Array(number=w194) -> (Boolean array=w196:bool[])
                n422 = Boolean To (0,1)(Boolean=w196) -> (0, 1=w193:i16[])
                n423 = Boolean To (0,1)(Boolean=w198) -> (0, 1=w197:i16[])
                n424 = case shown="79, 95" w191 {
                  tunnel: w193 -> [_ w206]
                  tunnel: w190 -> [_ w205]
                  frame 0, Default {
                  }
                  frame 79, 95 {
                    n425 = for {
                      tunnel: w206 -> [w211] mode=indexing
                      tunnel: w205 -> [w207]
                      i -> [w208]
                      stop <- w209 stop-if-true
                      n426 = Not Equal To 0?(x=w211) -> (x != 0?=w210:bool)
                      n427 = case shown="2" w208 {
                        tunnel: w210 -> [w212 w213 w214]
                        frame 0, Default {
                          "Ambient Sensor temp" <- w212
                        }
                        frame 1 {
                          "Ambient Over temp" <- w213
                        }
                        frame 2 {
                          "Hall Sensor Fault" <- w214
                        }
                      }
                      n428 = Equal?(x=w208, y=w207) -> (x = y?=w209:bool)
                    }
                  }
                }
                n429 = for {
                  tunnel: w197 -> [w216] mode=indexing
                  i -> [w217]
                  n430 = Not Equal To 0?(x=w216) -> (x != 0?=w215:bool)
                  n431 = case shown="0, Default" w217 {
                    tunnel: w215 -> [w218 w219 w220 w221 w222 w223 w224 w225]
                    frame 0, Default {
                      "Drive Sensor temp Failure" <- w218
                    }
                    frame 1 {
                      "Drive Over temperature" <- w219
                    }
                    frame 2 {
                      "Motor Sensor temp Fauilre" <- w220
                    }
                    frame 3 {
                      "Motor Over temperature" <- w221
                    }
                    frame 4 {
                      "Derated drive temp" <- w222
                    }
                    frame 5 {
                      "Under voltage/Over voltage" <- w223
                    }
                    frame 6 {
                      "Commutation err" <- w224
                    }
                    frame 7 {
                      "Speed error" <- w225
                    }
                  }
                }
              }
              frame 417474367, 417474383, 417474399 {
                w242 = "."
                # "Frame ID\n0x18E2273F"
                n432 = Index Array(array=w259, index #1=0 ("index")) -> (element #1=w257:u8, element #2=w255:u8, element #3=w236:u8, element #4=w237:u8, element #5=w238:u8, element #6=w239:u8)  [unwired: 5 in]
                n433 = Split Number(x=w238) -> (hi(x)=w250:u8, lo(x)=w249:u8)
                n434 = Split Number(x=w239) -> (hi(x)=w248:u8, lo(x)=w247:u8)
                n435 = Join Numbers(hi=w237, lo=w236) -> ((hi.lo)=w228:u16)
                n436 = Number To Hexadecimal String(2:w228) -> (0:w229:string)  [unwired: 1 in]
                n437 = Number To Decimal String(number=w250) -> (decimal integer string=w246:string)  [unwired: 1 in]
                n438 = Number To Decimal String(number=w249) -> (decimal integer string=w245:string)  [unwired: 1 in]
                n439 = Number To Decimal String(number=w248) -> (decimal integer string=w244:string)  [unwired: 1 in]
                n440 = Number To Decimal String(number=w247) -> (decimal integer string=w243:string)  [unwired: 1 in]
                n441 = Hexadecimal String To Number(string=w229) -> (number=w230:u32)  [unwired: 2 in, 1 out]
                n442 = To Double Precision Float(number=w230) -> (double precision float=w227:dbl)
                n443 = Number To Hexadecimal String(2:w255) -> (0:w253:string)  [unwired: 1 in]
                n444 = To Double Precision Float(number=w257) -> (double precision float=→"Motor Phase Current RMS":dbl)
                n445 = Multiply(x=w227, y=u16 1) -> (x*y=w234:dbl)
                n446 = Concatenate Strings(w246, w242, w245, w242, w244, w242, w243) -> (→"Driver Version":string)
                n447 = To Double Precision Float(number=w234) -> (double precision float=w233:dbl)
                "Motor Phase Current" <- w233
                n448 = Hexadecimal String To Number(string=w253) -> (number=w254:u32)  [unwired: 2 in, 1 out]
                n449 = To Double Precision Float(number=w254) -> (double precision float=w252:dbl)
                n450 = Subtract(x=w252, y=50.0) -> (x-y=→"Ambient Temperature":dbl)
                n451 = property on="Graph Plot" class="Bool (strict)"() -> ("Value"=w226:bool)  [unwired: 2 in, 2 out]
                n452 = case shown="True" w226 {
                  tunnel: w232 -> [w260 w263]
                  tunnel: [w260 w262] -> w231
                  tunnel: w233 -> [_ w261]
                  frame False {
                  }
                  frame True {
                    n453 = property on="Waveform Chart" class="WFChart (strict)"("Value"=w261) -> ()  [unwired: 2 in, 2 out]
                    n454 = Build Array (concatenate)(w261, w263) -> (w262:dbl[])
                  }
                }
              }
            }
            "Array 2" <- w130
          }
        }
      }
      frame "Stop" {
        n455 = Release Queue(queue=w1076, error in (no error)=w1078) -> (error out=w1077:errorcluster)  [unwired: 1 in, 2 out]
        n456 = flat-sequence {
          tunnel: w1075 -> [w1079]
          tunnel: [TRUE ("Stop")] -> w1074
          frame #0 {
            w1085 = u8[] [1, 0, 0, 0, 0, 0, 0, 0] ("Data 2")
            w1087 = u8 0 items=["STATUS"=128, "EXTENDED"=2, "RTR"=1, "DATA MSG"=0] ("MSGTYPE")
            w1092 = u8 1 items=["Standart flag", "Extern flag"] ("Format")
            w1091 = u8 0 items=["Data flag", "Remote flag"] ("Type")
            n457 = property on="Serial Status" class="Bool (strict)"() -> ("Value"=w1080:bool)  [unwired: 2 in, 2 out]
            n458 = property on="UUT" class="DigNum (strict)"() -> ("Value"=w1082:u8)  [unwired: 2 in, 2 out]
            n459 = case shown="True" w1080 {
              frame False {
              }
              frame True {
                n460 = property on="VISA resource name" class="VISAName"() -> ("Value"=w1103:refnum<visa-resource-name>)  [unwired: 2 in, 2 out]
                n461 = VISA Close(VISA resource name=w1103) -> ()  [unwired: 1 in, 1 out]
              }
            }
            n462 = case shown="95, Default" w1082 {
              tunnel: [u32 417357607 u32 417349415 u32 417345319] -> w1081
              frame 95, Default {
              }
              frame 63 {
              }
              frame 47 {
              }
            }
            n463 = property on="Graph Button" class="Bool (strict)"("Value"=FALSE ("Graph Button")) -> ()  [unwired: 2 in, 2 out]
            n464 = Array Size(array=w1085) -> (size(s)=w1090:i32)
            n465 = To Unsigned Byte Integer(number=w1090) -> (unsigned 8bit integer=w1088:u8)
            n466 = Bundle By Name(cluster=T10 {"ID"=0, "MSGTYPE"=0, "LEN"=0, "aDATA"=[]} ("MsgTX 2"), "ID"=w1081, "MSGTYPE"=w1087, "LEN"=w1088, "aDATA"=w1085) -> (w1086:T10)
            n467 = call "CANAnalData.vi"("ID"=w1081, "Data"=w1085, "Config"=w1079) -> ()  [unwired: 4 in, 5 out]
            n468 = call "Array Data to Single Num in Hex.vi"("aDATA"=w1085) -> ("Numeric"=w1084:u64)  [unwired: 10 in]
            n469 = property on="Data Send" class="DigNum (strict)"("Value"=w1084) -> ()  [unwired: 2 in, 2 out]
            n470 = Unbundle By Name(w1086) -> ("ID"=w1100:u32, "LEN"=w1101:u8, "aDATA"=w1102:u8[])  [unwired: 1 out]
            n471 = property class="Clust (strict)"(reference=w1079) -> ("Value"=w1099:T8)  [unwired: 1 in, 2 out]
            n472 = Bundle By Name(cluster=T14 {"ID"=0, "TimeStamp"=0, "TimeFlag"=0, "SendType"=0, "RemoteFlag"=0, "ExternFlag"=0, "DataLen"=0, "Data"=[], "Reserved"=[]} ("Send"), "ID"=w1100, "RemoteFlag"=w1091, "ExternFlag"=w1092, "DataLen"=w1101, "Data"=w1102) -> (w1097:T14)
            n473 = Unbundle By Name(w1099) -> ("DevType"=w1093:T2, "DevIndex"=w1094:u32, "CanIndex"=w1095:T3)
            n474 = Build Array(w1097) -> (w1096:T14[])
            n475 = call "VCI_Transmit.vi"("Buffer"=w1096, "CANIndex"=w1095, "DevIndex"=w1094, "DevType"=w1093) -> ()  [unwired: 1 in, 7 out]
          }
          frame #1 {
          }
        }
      }
    }
  }
  n476 = disable-structure shown="Disabled" {
    frame Disabled {
      n477 = control-ref of="Config_CANAT"() -> ()  [unwired: 1 out]
      n478 = control-ref of="UUT"() -> ()  [unwired: 1 out]
    }
    frame Enabled {
    }
  }
